vi "信号光谱6.vi"() -> ()   [LabVIEW 2018]
uses:
  <vilib>/Utility/NIReport.llb/Report Type.ctl
  <vilib>/Utility/file.llb/Write Delimited Spreadsheet (DBL).vi
  <vilib>/Instr/_visa.llb/VISA Configure Serial Port (Instr).vi
  <vilib>/addons/_office/excel.llb/Excel Get Data ([str]).vi
  <vilib>/Utility/NIReport.llb/NI_report.lvclass
  <vilib>/Analysis/NI_AALBase.lvlib
  <vilib>/ptbypt/NI_PtbyPt.lvlib
  <vilib>/Utility/NIReport.llb/NI_ReportGenerationCore.lvlib
  <vilib>/addons/_office/NI_ReportGenerationToolkit.lvlib
  <vilib>/Utility/NIReport.llb/Excel/NI_Excel.lvclass
panel:
  out "angle":dbl
  out "图片地址":string
  in  "开光时间/ms":u32=500
  out "最终存储路径 2":path
  out "照明光error out":errorcluster
  out "照明光":bool
  in  "stop bits (10: 1 bit)":u16(ring)=10 items=["1.0"=10, "1.5"=15, "2.0"=20]
  in  "parity (0:none)":enum16{"None", "Odd", "Even", "Mark", "Space"}(ring)
  in  "data bits (8)":u16=8 min=5 max=8 step=1
  in  "baud rate":u32=9600 caption="baud rate (115200)" min=9600 max=115200
  in  "VISA resource name":refnum<visa-resource-name>="COM7"
  out "正在测量":bool
  in  "滤波阈值":dbl=1500.0 format="%#_13g"
  out "best fit":dbl[][](graph) caption="最佳拟合"
  out "范围内？":bool[](array[boolean])
  out "w":dbl
  out "xc":dbl
  out "拟合参数":dbl[](array[numeric])
  out "最终存储路径":path
  in  "停止程序":bool
  in  "上升下降沿/s":dbl format="%.2p"
  in  "延时/s":dbl format="%.2p"
  in  "占空比/%":dbl=3.0 format="%.2p"
  in  "高电平/V":dbl=4.0 format="%.2p"
  in  "频率/Hz":dbl=6000.0 format="%.3p"
  in  "低电平/V":dbl min=0.0 max=5.0 format="%.2p"
  out "configure error out":errorcluster
  in  "设置参数":bool
  out "output control error  4":errorcluster
  in  "低电平持续输出":bool
  in  "Output 1":bool
  out "output control error  5":errorcluster
  in  "测量高电平/V":dbl=4.0
  out "output control error":errorcluster
  in  "开始测量":bool
  in  "上升下降沿":i32(ring)=1 items=["上升沿", "下降沿"]
  in  "channel输出口":i32(ring) items=["Channel 1", "Channel 2"]
  in  "输出信号波形":u16(ring) items=["Pulse"]
  out "output control error":errorcluster
  out "Output":bool
  in  "VISA 信号发生器":refnum<visa-resource-name>="USB0::0x1AB1::0x0641::DG4E192200870::INSTR"
  out "Spectrum":cluster{"Y":dbl[], "Y":dbl[]}[](graph)
  out "波长范围":dbl[](array[numeric])
  in  "选项卡控件":enum32{"IHR 550", "CCD"}(tab)
  in  "Move To\nTarget Positions":bool
  out "Current UniqueID":string="Mono4"
  in  "Mono ID":string(combo)="Mono1"
  in  "Connect":bool
  out "Initialized JY":bool=TRUE
  in  "Force\nInitialization":bool
  in  "Target Grating":string(combo)="2"
  out "Current Description":string="1" caption="Description"
  out "Grating Index":i32=1
  out "Current Grating":dbl=1200.0
  out "Units":string="nm"
  out "Current WL":dbl=897.9988
  out "Exit Mirror\nPosition":i32(ring)=2 items=["EntranceMirror", "ExitMirror", "Front", "Side"]
  out "Entrance Mirror\nPosition":i32(ring)=2 items=["EntranceMirror", "ExitMirror", "Front", "Side"]
  out "Units 2":string="mm"
  out "Front Entrance":dbl
  in  "Target WL":dbl=2670.0
  in  "Exit Mirror":u16(ring)=3 caption="Target Position Exit Mirror" items=["Front"=2, "Side"=3]
  in  "Entrance Mirror":u16(ring)=2 caption="Target Position\nEntrance Mirror" items=["Front"=2, "Side"=3]
  in  "Target\nFront Entrance":dbl=1.0
  in  "Commande tab":T1(tab)
  in  "Area Number to Display":i32
  in  "Reformat":bool
  in  "GAIN":u16(ring)=2 caption="Device Name" items=["High Light", "Best Dynamic Range", "High Sensitivity"]
  in  "ADC":u16(ring) caption="Device Name" items=["20 kHz       ", " 1 MHz       ", " 1 MHz Ultra "]
  in  "Number of Areas :":u16=1 min=1 step=1
  in  "Integration time (ms) :":i16=10000
  out "Uniques ID":u16(ring) items=["CCD1", "CCD2"]
  in  "Device Name":u16(ring) items=["Synapse CCD (Lateral)", "Synapse_IGA (Axial)"]
  in  "Signal type :":enum16{"TTL Rising Edge", "TTL Falling Edge"}(ring)=enum."TTL Falling Edge"
  in  "Trigger Type :":u16(ring) items=["On Start"=1, "Per Acquisition"=2]
  in  "trigSigTypeString":string
  in  "trigEventString":string
  in  "Enable InputTriggers :":bool
  in  "Number of Cleans":i32=1
  in  "MultiAcqShutterMode":i32(ring)=3 items=["Open For All Spectra"=1, "Open for Each Spectrum"=3]
  in  "Accumulations:":u16=10 min=1 step=1
  in  "Multi Accumulation mode:":bool
  out "Y Pixels:":i32=256
  out "DataSize":i32=1024
  out "X Pixels:":i32=1024
  out "Firmware\nVersion":string="V1.20 CCD_4000"
  out "initialized ?":bool=TRUE
  in  "Continuous":bool
  in  "CCD Busy":bool
  out "indicator":string="Ready !"
  in  "initialize":bool
  in  "ShutterOpen":bool=TRUE caption="Shutter enable"
  in  "Acquire":bool
  in  "Temperature":bool
  in  "Setup":bool
  out "Acq Time(ms)":u32=3401
  in  "Save Backlight":bool
  in  "cut backlight":bool
  out "backlight":bool=TRUE
  in  "是否拟合":bool
  in  "是否保存":bool
  in  "Close":bool=TRUE
  out "JYCCDLib.IJYCCDReqd":refnum<k7>
  out "areas :":i32[][](array[numeric])=[[1], [1], [1], [1024], [256], [1], [256]]
  in  "Constante de condition\n(Voir l'aide contextuelle)":bool
  out "temp graph":dbl(graph)=-134.538067
  out "ADC Number":i32[](array[numeric])=[0, 1, 2, 3, 4]
  out "Gain Number":i32[](array[numeric])=[10, 11, 12, 13, 8, 2]
  out "trigAddress":i32
  out "Data":i32[][](graph)
  out "error out":errorcluster
  out "Gratings":dbl[](array[numeric])=[1200.0, 300.0]
  out "Backlight":i32[][](graph)
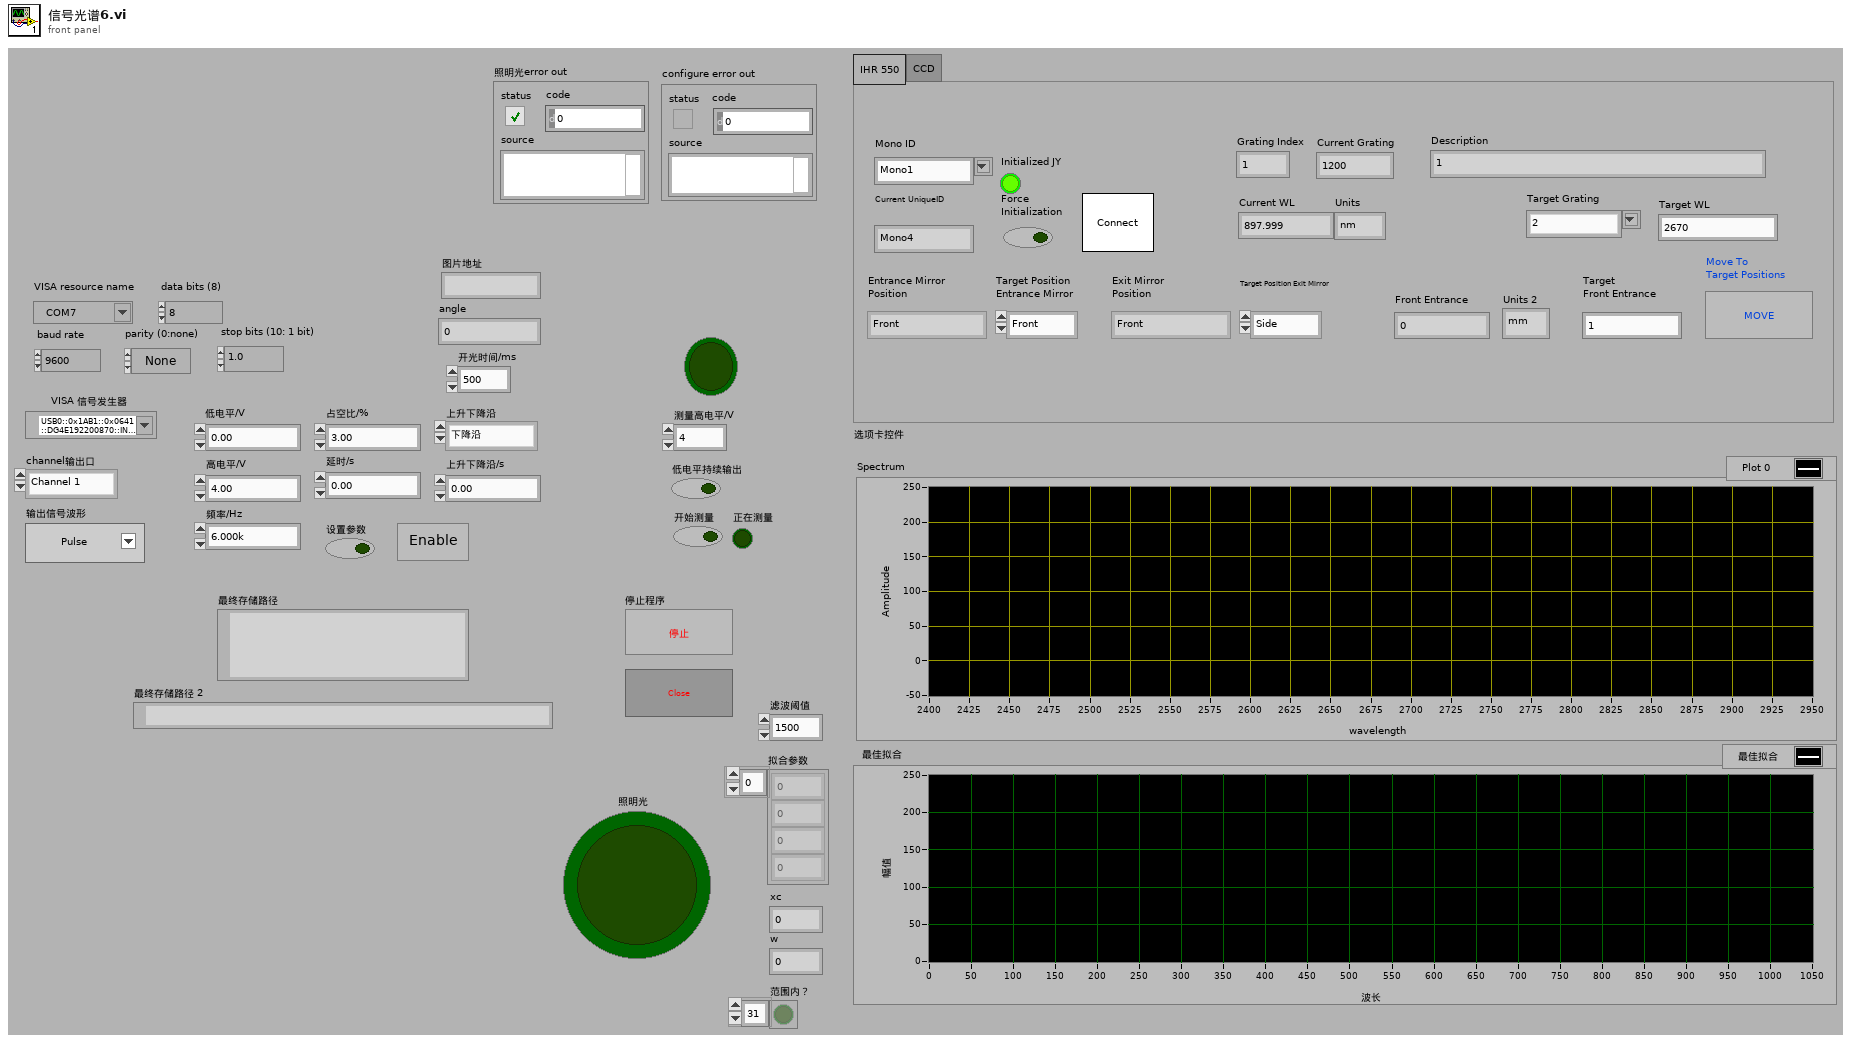
[diagram p1: front panel]
types:
  T1 = enum32{"Settings", "Trigger In", "Multi-Accu.", "Infos"}
  T2 = enum8{"Enabled", "Disabled", "Disabled and Grayed Out"}
  T3 = enum16{"maximized", "minimized", "normal", "no change"}
  T4 = typedef "NI_ReportGenerationCore.lvlib/Report Type.ctl" = enum16{"HTML", "Word", "Excel"}
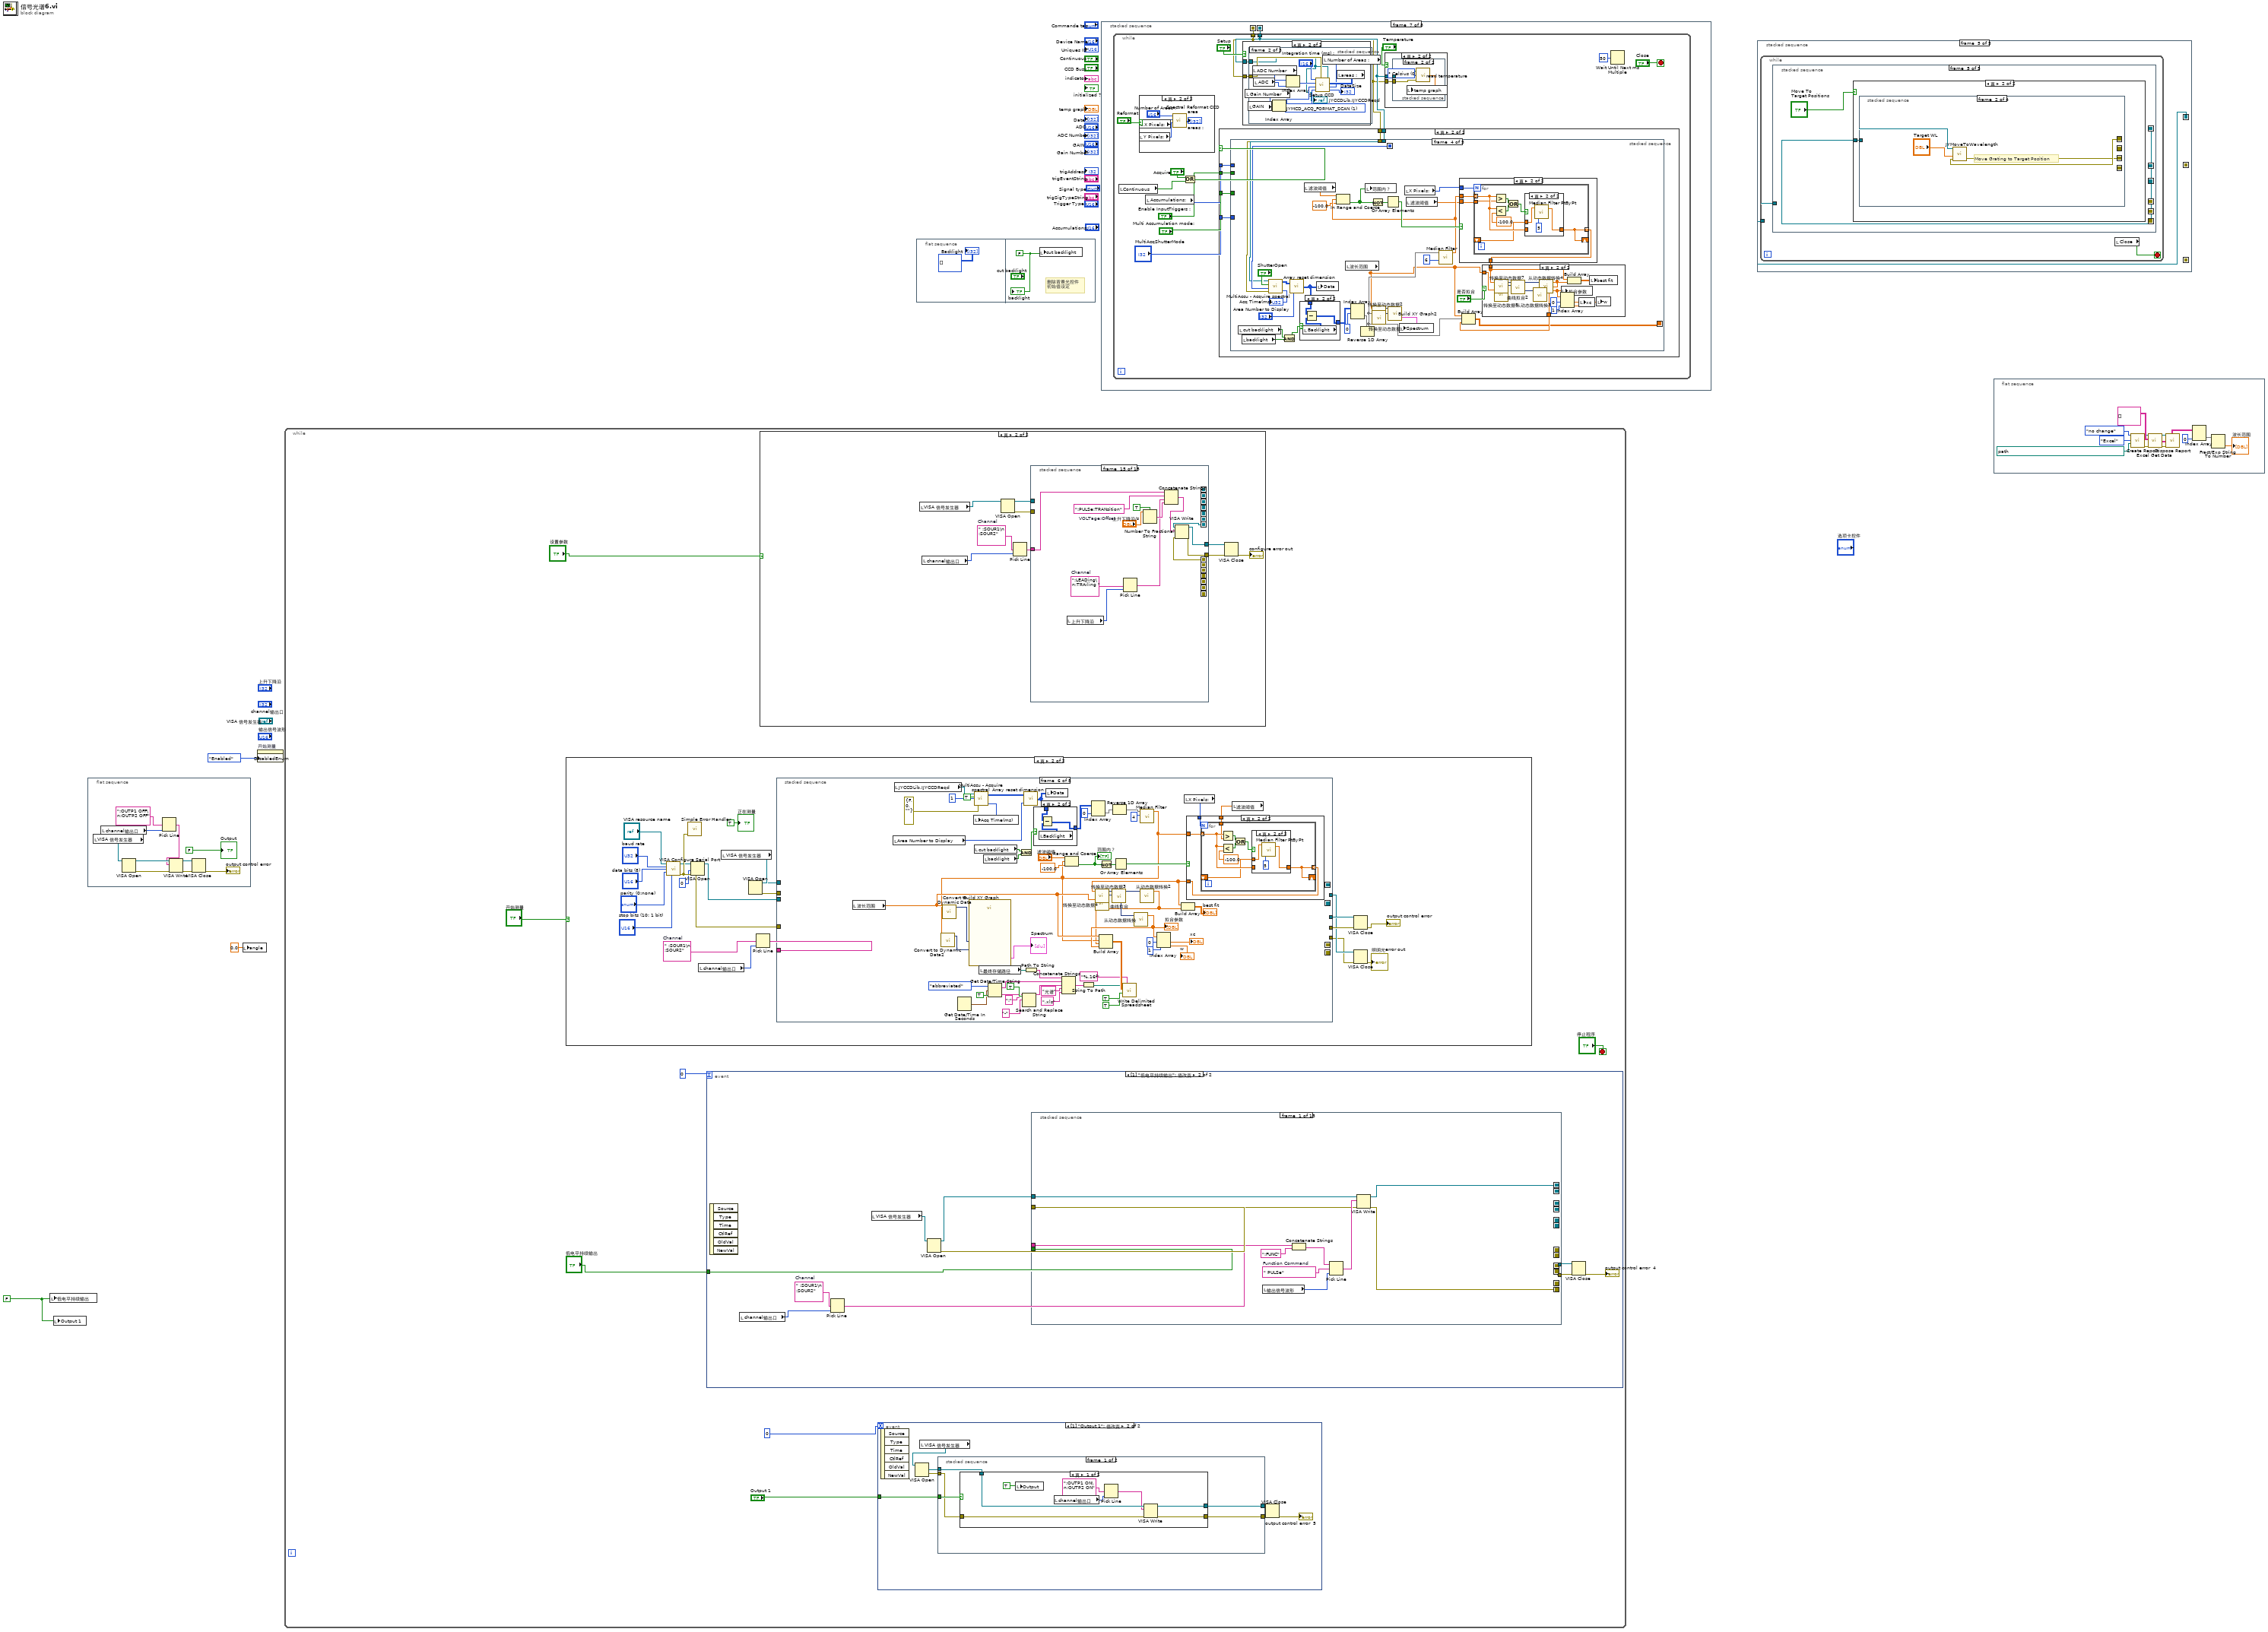
[diagram p0: block diagram]
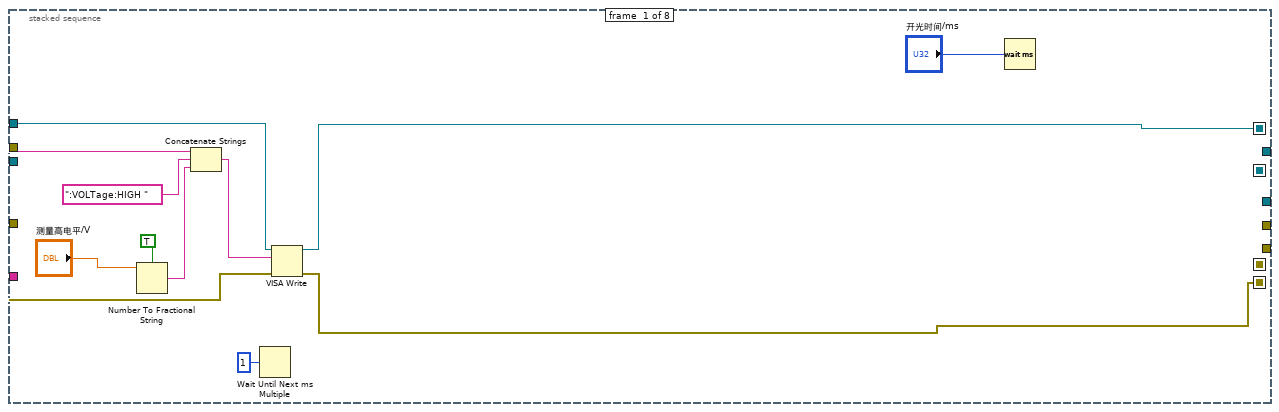
[diagram p3: hidden frame]
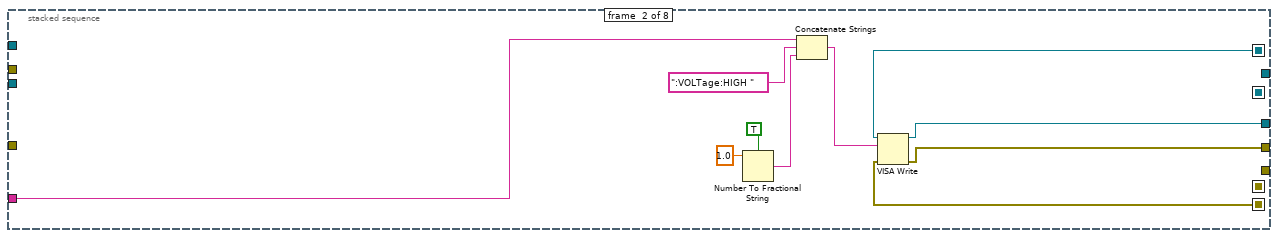
[diagram p4: hidden frame]
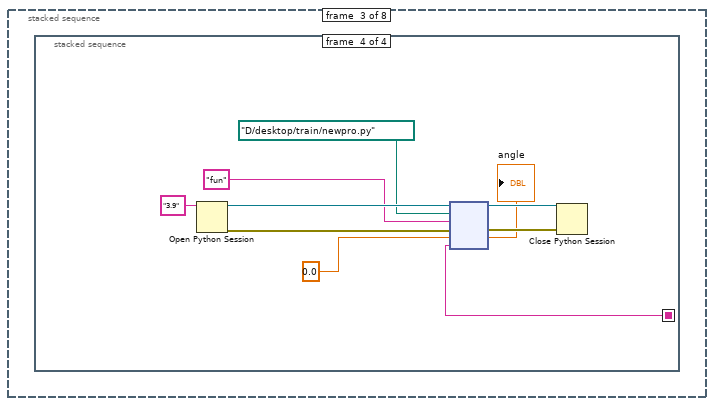
[diagram p5: hidden frame]
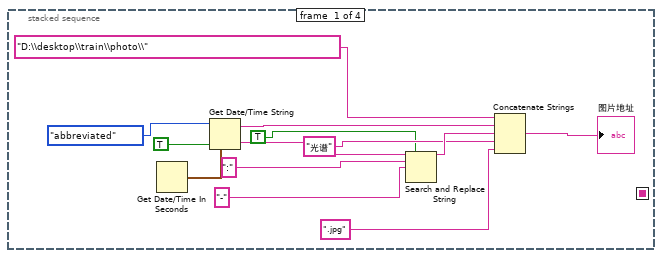
[diagram p6: hidden frame]
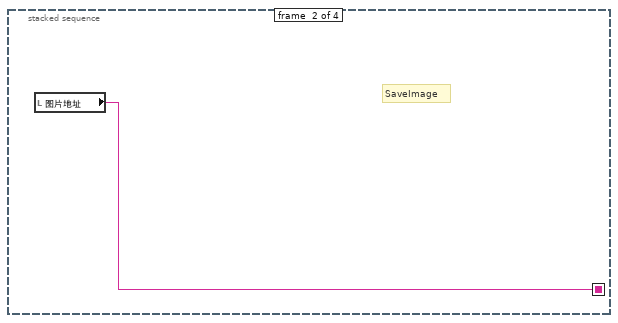
[diagram p7: hidden frame]
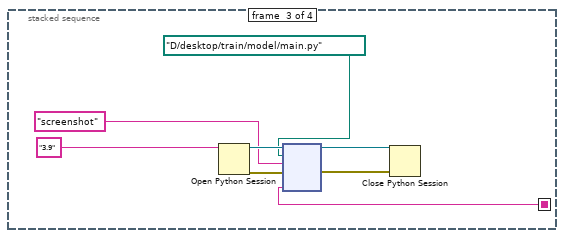
[diagram p8: hidden frame]
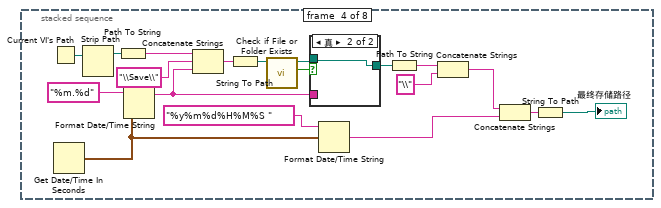
[diagram p9: hidden frame]
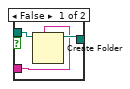
[diagram p10: hidden frame]
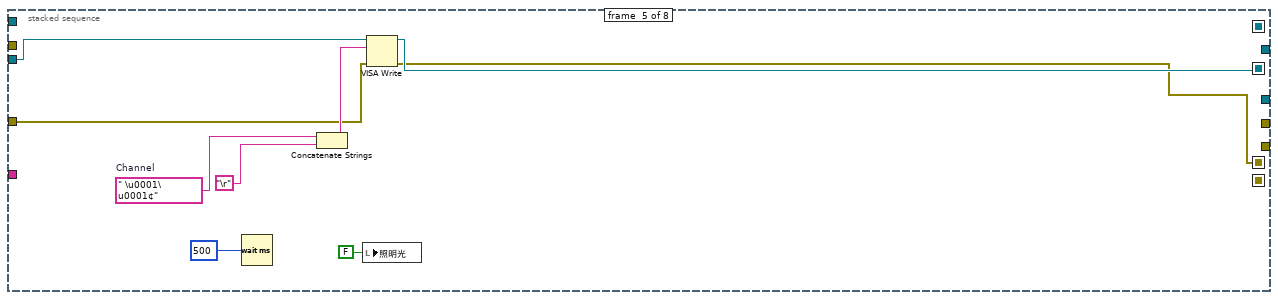
[diagram p11: hidden frame]
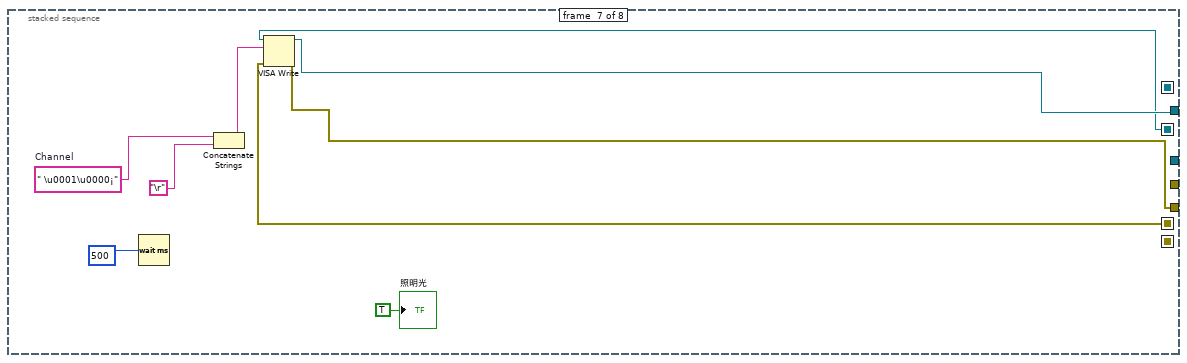
[diagram p15: hidden frame]
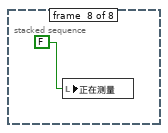
[diagram p16: hidden frame]
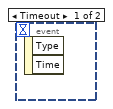
[diagram p17: hidden frame]
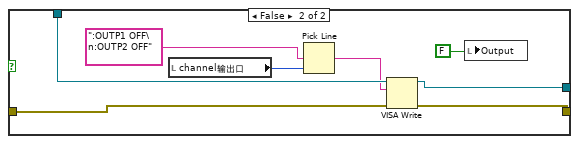
[diagram p18: hidden frame]
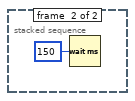
[diagram p19: hidden frame]
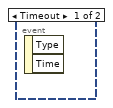
[diagram p20: hidden frame]
diagram:
  w2 = FALSE
  n1 = local write "低电平持续输出"(w2) -> ()
  n2 = local write "Output 1"(w2) -> ()
  n3 = flat-sequence {
    frame #0 {
      n4 = local read "VISA 信号发生器"() -> (w7:refnum<visa-resource-name>)
      n5 = local read "channel输出口"() -> (w5:i32)
      n6 = VISA Open(VISA resource name=w7) -> (VISA resource name=w13:refnum<visa-resource-name>, error out=w12:errorcluster)  [unwired: 4 in]
      n7 = Pick Line(multi-line string=":OUTP1 OFF\n:OUTP2 OFF" ("write buffer"), line index=w5) -> (output string=w4:string)  [unwired: 1 in]
      n8 = VISA Write(VISA resource name=w13, write buffer=w4, error in (no error)=w12) -> (VISA resource name out=w10:refnum<visa-resource-name>, error out=w9:errorcluster)  [unwired: 1 out]
      n9 = VISA Close(VISA resource name=w10, error in (no error)=w9) -> (error out=→"output control error":errorcluster)
      "Output" <- FALSE ("布尔")
    }
  }
  n10 = local write "angle"(0.0 ("angle")) -> ()
  n11 = property on="开始测量" class="Bool"("DisabledEnum"=T2."Enabled" ("禁用")) -> ()  [unwired: 2 in, 2 out]
  n12 = while {
    stop <- "停止程序" stop-if-true
    n13 = case shown="真" "开始测量" {
      frame False {
      }
      frame True {
        w36 = " :SOUR1\n :SOUR2"  # Channel
        n14 = call-poly "VISA Configure Serial Port"("VISA resource name"="VISA resource name", "baud rate (9600)"="baud rate", "data bits (8)"="data bits (8)", "parity (0:none)"="parity (0:none)", "stop bits (10: 1 bit)"="stop bits (10: 1 bit)") -> ("VISA resource name out"=w29:refnum<visa-resource-name>, "error out"=w30:errorcluster)  [unwired: 9 in]
        n15 = call <vilib>:"Simple Error Handler.vi"("error in (no error)"=w30) -> ()  [unwired: 4 in, 5 out]
        n16 = VISA Open(access mode=0, error in (no error)=w30, VISA resource name=w29) -> (VISA resource name=w22:refnum<visa-resource-name>, error out=w21:errorcluster)  [unwired: 2 in]
        n17 = local read "channel输出口"() -> (w37:i32)
        n18 = local read "VISA 信号发生器"() -> (w43:refnum<visa-resource-name>)
        n19 = VISA Open(VISA resource name=w43) -> (VISA resource name=w42:refnum<visa-resource-name>, error out=w41:errorcluster)  [unwired: 4 in]
        n20 = Pick Line(multi-line string=w36, line index=w37) -> (output string=w35:string)  [unwired: 1 in]
        n21 = stacked-sequence {
          seq-local: [w47 _ _ _ _ _ _ _] -> [_ w58 _ _ _ _ _ _]
          seq-local: [w46 _ _ _ _ _ _ _] -> [_ w57 _ _ _ _ _ _]
          seq-local: [_ _ _ _ w122 _ _ _] -> [_ _ _ _ _ _ w210 _]
          seq-local: [_ _ _ _ w121 _ _ _] -> [_ _ _ _ _ _ w213 _]
          tunnel: w42 -> [w50 _ _ _ _ _ _ _]
          tunnel: w41 -> [w49 _ _ _ _ _ _ _]
          tunnel: [_ w60 _ _ _ _ _ _] -> w40
          tunnel: [_ w59 _ _ _ _ _ _] -> w39
          tunnel: w35 -> [w51 w56 _ _ _ _ _ _]
          tunnel: w22 -> [_ _ _ _ w125 _ _ _]
          tunnel: w21 -> [_ _ _ _ w124 _ _ _]
          tunnel: [_ _ _ _ _ _ w212 _] -> w33
          tunnel: [_ _ _ _ _ _ w211 _] -> w32
          frame #0 {
            n22 = Number To Fractional String(use system decimal point (T)=TRUE ("使用系统小数点(T)"), number="测量高电平/V") -> (F-format string=w53:string)  [unwired: 2 in]
            n23 = Concatenate Strings ("连接字符串")(w51, ":VOLTage:HIGH ", w53) -> (w52:string)
            n24 = Wait Until Next ms Multiple(millisecond multiple=u32 1 ("毫秒倍数")) -> ()  [unwired: 1 out]
            n25 = VISA Write(VISA resource name=w50, write buffer=w52, error in (no error)=w49) -> (VISA resource name out=w47:refnum<visa-resource-name>, error out=w46:errorcluster)  [unwired: 1 out]
            n26 = Wait (ms)(milliseconds to wait="开光时间/ms") -> ()  [unwired: 1 out]
          }
          frame #1 {
            n27 = Number To Fractional String(use system decimal point (T)=TRUE ("使用系统小数点(T)"), number=1.0 ("数字")) -> (F-format string=w63:string)  [unwired: 2 in]
            n28 = Concatenate Strings ("连接字符串")(w56, ":VOLTage:HIGH ", w63) -> (w62:string)
            n29 = VISA Write(VISA resource name=w58, write buffer=w62, error in (no error)=w57) -> (VISA resource name out=w60:refnum<visa-resource-name>, error out=w59:errorcluster)  [unwired: 1 out]
          }
          frame #2 {
            n30 = stacked-sequence {
              seq-local: [_ w79 _ _] -> [_ _ w80 w88]
              frame #0 {
                n31 = Get Date/Time In Seconds() -> (seconds since 1Jan1904=w75:timestamp)
                n32 = Get Date/Time String(date format (0)=enum16{"short", "long", "abbreviated"}."abbreviated" ("日期格式(0)"), seconds (now)=w75, want seconds? (F)=TRUE ("需要秒？(F)")) -> (date string=w78:string, time string=w76:string)
                n33 = Search and Replace String(replace all?=TRUE ("替换全部？(F)"), input string=w76, search string=":" ("搜索字符串"), replace string="-" ("替换字符串(\"\")")) -> (result string=w77:string)  [unwired: 4 in, 3 out]
                n34 = Concatenate Strings("D:\\desktop\\train\\photo\\", w78, w77, "光谱" ("字符串"), ".jpg" ("字符串")) -> (→"图片地址":string)
              }
              frame #1 {
                # "SaveImage"
                n35 = local read "图片地址"() -> (w79:string)
              }
              frame #2 {
                n36 = Open Python Session(python version="3.9" ("Python version")) -> (session out=w87:refnum<k35>, error out=w85:errorcluster)  [unwired: 2 in]
                n37 = node(w87, path "D:/desktop/train/model/main.py" ("module path"), "screenshot" ("function name"), w85, w80) -> (w86:refnum<k35>, w84:errorcluster)  [unwired: 3 in, 2 out]
                n38 = Close Python Session(session in=w86, error in=w84) -> ()  [unwired: 1 out]
              }
              frame #3 {
                n39 = Open Python Session(python version="3.9" ("Python version")) -> (session out=w96:refnum<k35>, error out=w94:errorcluster)  [unwired: 2 in]
                n40 = node(w96, path "D:/desktop/train/newpro.py" ("module path"), "fun" ("function name"), w94, 0.0, w88) -> (w95:refnum<k35>, w93:errorcluster, →"angle":dbl)  [unwired: 1 in, 2 out]
                n41 = Close Python Session(session in=w95, error in=w93) -> ()  [unwired: 1 out]
              }
            }
          }
          frame #3 {
            n42 = Current VI's Path() -> (path=w103:path)
            n43 = Get Date/Time In Seconds() -> (seconds since 1Jan1904=w105:timestamp)
            n44 = Strip Path(path=w103) -> (stripped path=w104:path)  [unwired: 1 out]
            n45 = Path To String(path=w104) -> (string=w106:string)
            n46 = Format Date/Time String(time format string (%c)="%m.%d" ("时间格式字符串(%c)"), seconds (now)=w105) -> (date/time string=w112:string)  [unwired: 1 in]
            n47 = Concatenate Strings(w106, "\\Save\\" ("字符串"), w112) -> (w107:string)
            n48 = String To Path(string=w107) -> (path=w108:path)
            n49 = call <vilib>:"Check if File or Folder Exists.vi"("path"=w108) -> ("file or folder exists?"=w109:bool, "dup path"=w111:path)  [unwired: 8 in, 1 out]
            n50 = case shown="真" w109 {
              tunnel: [w119 w120] -> w110
              tunnel: w111 -> [w118 w120]
              tunnel: w112 -> [w117 _]
              frame False {
                n51 = Create Folder(prompt (Create Folder)=w117, path (use dialog)=w118) -> (created path=w119:path)  [unwired: 1 in, 2 out]
              }
              frame True {
              }
            }
            n52 = Format Date/Time String(time format string (%c)="%y%m%d%H%M%S " ("时间格式字符串(%c)"), seconds (now)=w105) -> (date/time string=w115:string)  [unwired: 1 in]
            n53 = Path To String(path=w110) -> (string=w113:string)
            n54 = Concatenate Strings(w113, "\\" ("字符串")) -> (w114:string)
            n55 = Concatenate Strings(w114, w115) -> (w102:string)
            n56 = String To Path(string=w102) -> (path=→"最终存储路径":path)
          }
          frame #4 {
            w126 = " \u0001\u0001¢"  # Channel
            n57 = Wait (ms)(milliseconds to wait=500) -> ()  [unwired: 1 out]
            n58 = Concatenate Strings(w126, "\r") -> (w127:string)
            n59 = local write "照明光"(FALSE ("照明光")) -> ()
            n60 = VISA Write(VISA resource name=w125, write buffer=w127, error in (no error)=w124) -> (VISA resource name out=w122:refnum<visa-resource-name>, error out=w121:errorcluster)  [unwired: 1 out]
          }
          frame #5 {
            n61 = local read "波长范围"() -> (w152:dbl[])
            n62 = local read "Area Number to Display"() -> (w162:i32)
            n63 = local read "JYCCDLib.IJYCCDReqd"() -> (w158:refnum<k7>)
            n64 = call "Convert to Dynamic Data"("Array"=w152) -> ("Dynamic Data Type"=w155:dynamicdata)  [unwired: 3 in]
            n65 = Get Date/Time In Seconds() -> (seconds since 1Jan1904=w171:timestamp)
            n66 = call "MultiAccu - Acquire spectral.vi"("error in"=errorcluster {"status"=FALSE, "code"=0, "source"=""}, "Accumulations:"=u16 1, "ShutterOpen"=TRUE, "JYCCDLib.IJYCCDReqd"=w158) -> ("Acq Time(ms)"=w164:u32, "Array Out"=w163:i32[][][])  [unwired: 1 out]
            n67 = local write "Acq Time(ms)"(w164) -> ()
            n68 = local read "cut backlight"() -> (w143:bool)
            n69 = local read "最终存储路径"() -> (w185:path)
            n70 = local read "backlight"() -> (w141:bool)
            n71 = Get Date/Time String(date format (0)=enum16{"short", "long", "abbreviated"}."abbreviated" ("日期格式(0)"), seconds (now)=w171, want seconds? (F)=TRUE ("需要秒？(F)")) -> (date string=w179:string, time string=w174:string)
            n72 = And(x=w143, y=w141) -> (x .and. y?=w142:bool)
            n73 = Search and Replace String(replace all?=TRUE ("替换全部？(F)"), input string=w174, search string=":" ("搜索字符串"), replace string="-" ("替换字符串(\"\")")) -> (result string=w178:string)  [unwired: 4 in, 3 out]
            n74 = call "Array reset dimension.vi"("Area Number"=w162, "Array In"=w163) -> ("Array Out"=w145:i32[][])
            n75 = Path To String(path=w185) -> (string=w168:string)
            n76 = case shown="真" w142 {
              tunnel: [w206 w208] -> w144
              tunnel: w145 -> [w206 w207]
              frame False {
              }
              frame True {
                n77 = local read "Backlight"() -> (w209:i32[][])
                n78 = Subtract(x=w207, y=w209) -> (x-y=w208:i32[][])
              }
            }
            n79 = local write "Data"(w145) -> ()
            n80 = Concatenate Strings(w168, w179, w178, "光谱" ("字符串"), ".xls" ("字符串")) -> (w183:string)
            n81 = String To Path(string=w183) -> (path=w184:path)
            n82 = Index Array(array=w144, index (row)=0 ("索引 (行)")) -> (element=w186:i32[])  [unwired: 1 in]
            n83 = call "转换至动态数据4"("Array"=w152) -> ("Dynamic Data Type"=w151:dynamicdata)  [unwired: 3 in]
            n84 = Reverse 1D Array(array=w186) -> (reversed array=w187:i32[])
            n85 = call <vilib>:"Median Filter.vi"("left rank"=4, "X"=w187) -> ("Filtered X"=w136:dbl[])  [unwired: 8 in, 1 out]
            n86 = call "Convert to Dynamic Data2"("Array"=w136) -> ("Dynamic Data Type"=w154:dynamicdata)  [unwired: 3 in]
            n87 = call "Build XY Graph"("Y Input"=w154, "X Input"=w155) -> ("XY Graph"=→"Spectrum":cluster{"Y":dbl[], "Y":dbl[]}[])  [unwired: 8 in, 1 out]
            n88 = In Range and Coerce(upper limit="滤波阈值", x=w136, lower limit=-100.0) -> (In Range?=w135:bool[])  [unwired: 1 out]
            "范围内？" <- w135
            n89 = Not(x=w135) -> (.not. x?=w134:bool[])
            n90 = Or Array Elements(Boolean array=w134) -> (logical OR=w138:bool)
            n91 = local read "X Pixels:"() -> (w137:i32)
            n92 = local read "滤波阈值"() -> (w130:dbl)
            n93 = case shown="真" w138 {
              tunnel: w137 -> [_ w193]
              tunnel: w136 -> [w189 w192]
              tunnel: [w189 w191] -> w133
              tunnel: w130 -> [_ w190]
              frame False {
              }
              frame True {
                n94 = for {
                  N: w193 -> [_]
                  tunnel: w192 -> [w197] mode=indexing
                  tunnel: [w196] -> w191 mode=indexing
                  shift-right: [w196] -> _
                  shift-left: _ -> [w195]
                  tunnel: w190 -> [w194]
                  n95 = Greater?(x=w197, y=w194) -> (0:w199:bool)
                  n96 = Less?(x=w197, y=-100.0) -> (x < y?=w200:bool)
                  n97 = Or(x=w199, y=w200) -> (x .or. y?=w198:bool)
                  n98 = case shown="真" w198 {
                    tunnel: w197 -> [w202 _]
                    tunnel: [w202 w204] -> w196
                    tunnel: w195 -> [_ w205]
                    frame False {
                    }
                    frame True {
                      n99 = call <vilib>:"Median Filter PtByPt.vi"("rank"=5, "x"=w205) -> ("Filtered x"=w204:dbl)  [unwired: 2 in, 1 out]
                    }
                  }
                }
              }
            }
            n100 = call "转换至动态数据3"("Array"=w133) -> ("Dynamic Data Type"=w153:dynamicdata)  [unwired: 3 in]
            n101 = call "曲线拟合"("Locations"=w151, "Signals"=w153) -> ("best fit"=w157:dynamicdata, "non-linear coefficients"=w156:dynamicdata)  [unwired: 5 in, 3 out]
            n102 = call "从动态数据转换"("Dynamic Data Type"=w156) -> ("Array"=w148:dbl[])  [unwired: 3 in]
            "拟合参数" <- w148
            n103 = call "从动态数据转换2"("Dynamic Data Type"=w157) -> ("Array"=w132:dbl[])  [unwired: 3 in]
            n104 = Build Array(w152, w136, w132, w148) -> (w188:dbl[][])
            n105 = call-poly <vilib>:"Write Delimited Spreadsheet.vi"("file path (dialog if empty)"=w184, "format (%.3f)"="%.16f", "2D data"=w188, "append to file? (new file:F)"=TRUE ("append to file? (F)"), "transpose? (no:F)"=TRUE ("transpose? (F)")) -> ()  [unwired: 9 in, 2 out]
            n106 = Index Array(array=w148, index #1=0 ("索引"), index #2=1 ("索引")) -> (element #1=→"xc":dbl, element #2=→"w":dbl)
            n107 = Build Array(w133, w132) -> (→"best fit":dbl[][])
          }
          frame #6 {
            w215 = " \u0001\u0000¡"  # Channel
            n108 = Wait (ms)(milliseconds to wait=500) -> ()  [unwired: 1 out]
            n109 = Concatenate Strings(w215, "\r") -> (w216:string)
            n110 = VISA Write(VISA resource name=w210, write buffer=w216, error in (no error)=w213) -> (VISA resource name out=w212:refnum<visa-resource-name>, error out=w211:errorcluster)  [unwired: 1 out]
            "照明光" <- TRUE ("照明光")
          }
          frame #7 {
            n111 = local write "正在测量"(FALSE) -> ()
          }
        }
        n112 = VISA Close(VISA resource name=w40, error in (no error)=w39) -> (error out=→"output control error":errorcluster)
        n113 = VISA Close(VISA resource name=w33, error in (no error)=w32) -> (error out=→"照明光error out":errorcluster)
        "正在测量" <- TRUE
      }
    }
    n114 = event shown="[1] \"低电平持续输出\": 值改变" {
      selector: _ -> [_ _]
      dyn-events: _ -> [_ _]
      timeout: u32 0 ("Time") -> [_ _]
      tunnel: "低电平持续输出" -> [_ w249]
      event Timeout {
        n115 = event-data() -> ()  [unwired: 1 in, 2 out]
      }
      event "低电平持续输出": Value Change {
        w253 = " :SOUR1\n :SOUR2"  # Channel
        n116 = event-data() -> ()  [unwired: 1 in, 6 out]
        n117 = local read "channel输出口"() -> (w254:i32)
        n118 = Pick Line(multi-line string=w253, line index=w254) -> (output string=w252:string)  [unwired: 1 in]
        n119 = local read "VISA 信号发生器"() -> (w257:refnum<visa-resource-name>)
        n120 = VISA Open(VISA resource name=w257) -> (VISA resource name=w256:refnum<visa-resource-name>, error out=w255:errorcluster)  [unwired: 4 in]
        n121 = stacked-sequence {
          seq-local: [w263 _ _ _ _ _ _ _ _ _ _ _ _] -> [_ _ w278 _ _ _ _ _ _ _ _ _ _]
          seq-local: [w262 _ _ _ _ _ _ _ _ _ _ _ _] -> [_ _ w277 _ _ _ _ _ _ _ _ _ _]
          seq-local: [_ _ w276 _ _ _ _ _ _ _ _ _ _] -> [_ _ _ _ w281 _ _ _ _ _ _ _ _]
          seq-local: [_ _ w275 _ _ _ _ _ _ _ _ _ _] -> [_ _ _ _ w282 _ _ _ _ _ _ _ _]
          seq-local: [_ _ _ _ w290 _ _ _ _ _ _ _ _] -> [_ _ _ _ _ _ w301 _ _ _ _ _ _]
          seq-local: [_ _ _ _ w289 _ _ _ _ _ _ _ _] -> [_ _ _ _ _ _ w300 _ _ _ _ _ _]
          seq-local: [_ _ _ _ _ _ w294 _ _ _ _ _ _] -> [_ _ _ _ _ _ _ _ w304 _ _ _ _]
          seq-local: [_ _ _ _ _ _ w293 _ _ _ _ _ _] -> [_ _ _ _ _ _ _ _ w303 _ _ _ _]
          seq-local: [_ _ _ _ _ _ _ _ w307 _ _ _ _] -> [_ _ _ _ _ _ _ _ _ _ w318 _ _]
          seq-local: [_ _ _ _ _ _ _ _ w306 _ _ _ _] -> [_ _ _ _ _ _ _ _ _ _ w317 _ _]
          seq-local: [_ _ _ _ _ _ _ _ _ _ w315 _ _] -> [_ _ _ _ _ _ _ _ _ _ _ _ w332]
          seq-local: [_ _ _ _ _ _ _ _ _ _ w314 _ _] -> [_ _ _ _ _ _ _ _ _ _ _ _ w331]
          tunnel: w256 -> [w268 _ _ _ _ _ _ _ _ _ _ _ _]
          tunnel: w255 -> [w261 _ _ _ _ _ _ _ _ _ _ _ _]
          tunnel: w252 -> [w260 _ w274 _ w287 _ w298 _ w308 _ w321 _ _]
          tunnel: [_ _ _ _ _ _ _ _ _ _ _ _ w330] -> w251
          tunnel: [_ _ _ _ _ _ _ _ _ _ _ _ w328] -> w250
          tunnel: w249 -> [_ _ _ _ _ _ _ _ _ _ _ _ w329]
          frame #0 {
            w265 = " PULSe"  # Function Command
            n122 = local read "输出信号波形"() -> (w259:u16)
            n123 = Concatenate Strings(w260, ":FUNC" ("string (\"\")")) -> (w266:string)
            n124 = Pick Line(string ("")=w266, multi-line string=w265, line index=w259) -> (output string=w264:string)
            n125 = VISA Write(VISA resource name=w268, write buffer=w264, error in (no error)=w261) -> (VISA resource name out=w263:refnum<visa-resource-name>, error out=w262:errorcluster)  [unwired: 1 out]
          }
          frame #1 {
            n126 = Wait (ms)(milliseconds to wait=u32 150) -> ()  [unwired: 1 out]
          }
          frame #2 {
            n127 = Number To Fractional String(use system decimal point (T)=TRUE ("使用系统小数点(T)"), number=1.0 ("数字")) -> (F-format string=w272:string)  [unwired: 2 in]
            n128 = Concatenate Strings ("连接字符串")(w274, ":VOLTage：HIGH ", w272) -> (w271:string)
            n129 = VISA Write(VISA resource name=w278, write buffer=w271, error in (no error)=w277) -> (VISA resource name out=w276:refnum<visa-resource-name>, error out=w275:errorcluster)  [unwired: 1 out]
          }
          frame #3 {
            n130 = Wait (ms)(milliseconds to wait=u32 150) -> ()  [unwired: 1 out]
          }
          frame #4 {
            # "1 电压偏置"
            n131 = Number To Fractional String(use system decimal point (T)=TRUE ("使用系统小数点(T)"), number=0.0 ("数字")) -> (F-format string=w285:string)  [unwired: 2 in]
            n132 = Concatenate Strings(w287, ":VOLTage:LOW ", w285) -> (w286:string)
            n133 = VISA Write(VISA resource name=w281, write buffer=w286, error in (no error)=w282) -> (VISA resource name out=w290:refnum<visa-resource-name>, error out=w289:errorcluster)  [unwired: 1 out]
          }
          frame #5 {
            n134 = Wait (ms)(milliseconds to wait=u32 150) -> ()  [unwired: 1 out]
          }
          frame #6 {
            n135 = local read "channel输出口"() -> (w296:i32)
            n136 = Pick Line(multi-line string=":OUTP1:IMPedance \n:OUTP2:IMPedance " ("write buffer"), line index=w296) -> (output string=w295:string)  [unwired: 1 in]
            n137 = Concatenate Strings ("连接字符串")(w298, w295, "INFINITY") -> (w299:string)
            n138 = VISA Write(VISA resource name=w301, write buffer=w299, error in (no error)=w300) -> (VISA resource name out=w294:refnum<visa-resource-name>, error out=w293:errorcluster)  [unwired: 1 out]
          }
          frame #7 {
            n139 = Wait (ms)(milliseconds to wait=u32 150) -> ()  [unwired: 1 out]
          }
          frame #8 {
            n140 = Number To Fractional String(use system decimal point (T)=TRUE ("使用系统小数点(T)"), number=0.0 ("数字")) -> (F-format string=w311:string)  [unwired: 2 in]
            n141 = Concatenate Strings(w308, ":PULSe:DELay ", w311) -> (w309:string)
            n142 = VISA Write(VISA resource name=w304, write buffer=w309, error in (no error)=w303) -> (VISA resource name out=w307:refnum<visa-resource-name>, error out=w306:errorcluster)  [unwired: 1 out]
          }
          frame #9 {
            n143 = Wait (ms)(milliseconds to wait=u32 150) -> ()  [unwired: 1 out]
          }
          frame #10 {
            w322 = ":LEADing\n:TRAiling "  # Channel
            w326 = ":PULSe:TRANsition"  # VOLTage:Offset
            n144 = local read "上升下降沿"() -> (w323:i32)
            n145 = Pick Line(multi-line string=w322, line index=w323) -> (output string=w319:string)  [unwired: 1 in]
            n146 = Number To Fractional String(use system decimal point (T)=TRUE ("使用系统小数点(T)"), number=0.0 ("数字")) -> (F-format string=w320:string)  [unwired: 2 in]
            n147 = Concatenate Strings(w321, w326, w319, w320) -> (w324:string)
            n148 = VISA Write(VISA resource name=w318, write buffer=w324, error in (no error)=w317) -> (VISA resource name out=w315:refnum<visa-resource-name>, error out=w314:errorcluster)  [unwired: 1 out]
          }
          frame #11 {
            n149 = Wait (ms)(milliseconds to wait=u32 150) -> ()  [unwired: 1 out]
          }
          frame #12 {
            n150 = case shown="假" w329 {
              tunnel: w332 -> [w340 w341]
              tunnel: [w339 w348] -> w328
              tunnel: w331 -> [w338 w346]
              tunnel: [w337 w347] -> w330
              frame True {
                n151 = local write "Output"(TRUE ("布尔")) -> ()
                n152 = local read "channel输出口"() -> (w334:i32)
                n153 = Pick Line(multi-line string=":OUTP1 ON\n:OUTP2 ON" ("write buffer"), line index=w334) -> (output string=w333:string)  [unwired: 1 in]
                n154 = VISA Write(VISA resource name=w340, write buffer=w333, error in (no error)=w338) -> (VISA resource name out=w337:refnum<visa-resource-name>, error out=w339:errorcluster)  [unwired: 1 out]
              }
              frame False {
                n155 = local read "channel输出口"() -> (w343:i32)
                n156 = Pick Line(multi-line string=":OUTP1 OFF\n:OUTP2 OFF" ("write buffer"), line index=w343) -> (output string=w342:string)  [unwired: 1 in]
                n157 = VISA Write(VISA resource name=w341, write buffer=w342, error in (no error)=w346) -> (VISA resource name out=w347:refnum<visa-resource-name>, error out=w348:errorcluster)  [unwired: 1 out]
                n158 = local write "Output"(FALSE ("布尔")) -> ()
              }
            }
          }
        }
        n159 = VISA Close(VISA resource name=w251, error in (no error)=w250) -> (error out=→"output control error  4":errorcluster)
      }
    }
    n160 = case shown="真" "设置参数" {
      frame False {
      }
      frame True {
        w354 = " :SOUR1\n :SOUR2"  # Channel
        n161 = local read "VISA 信号发生器"() -> (w350:refnum<visa-resource-name>)
        n162 = local read "channel输出口"() -> (w349:i32)
        n163 = VISA Open(VISA resource name=w350) -> (VISA resource name=w356:refnum<visa-resource-name>, error out=w357:errorcluster)  [unwired: 4 in]
        n164 = Pick Line(multi-line string=w354, line index=w349) -> (output string=w353:string)  [unwired: 1 in]
        n165 = stacked-sequence {
          seq-local: [w362 _ _ _ _ _ _ _ _ _ _ _ _ _ _] -> [_ _ w377 _ _ _ _ _ _ _ _ _ _ _ _]
          seq-local: [w361 _ _ _ _ _ _ _ _ _ _ _ _ _ _] -> [_ _ w376 _ _ _ _ _ _ _ w415 _ _ _ _]
          seq-local: [_ _ w375 _ _ _ _ _ _ _ _ _ _ _ _] -> [_ _ _ _ w386 _ _ _ _ _ _ _ _ _ _]
          seq-local: [_ _ w374 _ _ _ _ _ _ _ _ _ _ _ _] -> [_ _ _ _ w385 _ _ _ _ _ _ _ _ _ _]
          seq-local: [_ _ _ _ w384 _ _ _ _ _ _ _ _ _ _] -> [_ _ _ _ _ _ w392 _ _ _ _ _ _ _ _]
          seq-local: [_ _ _ _ w381 _ _ _ _ _ _ _ _ _ _] -> [_ _ _ _ _ _ w391 _ _ _ _ _ _ _ _]
          seq-local: [_ _ _ _ _ _ w399 _ _ _ _ _ _ _ _] -> [_ _ _ _ _ _ _ _ w410 _ _ _ _ _ _]
          seq-local: [_ _ _ _ _ _ w398 _ _ _ _ _ _ _ _] -> [_ _ _ _ _ _ _ _ w409 _ _ _ _ _ _]
          seq-local: [_ _ _ _ _ _ _ _ w403 _ _ _ _ _ _] -> [_ _ _ _ _ _ _ _ _ _ w416 _ _ _ _]
          seq-local: [_ _ _ _ _ _ _ _ w402 _ _ _ _ _ _] -> [_ _ _ _ _ _ _ _ _ _ _ _ _ _ _]
          seq-local: [_ _ _ _ _ _ _ _ _ _ w412 _ _ _ _] -> [_ _ _ _ _ _ _ _ _ _ _ _ w426 _ _]
          seq-local: [_ _ _ _ _ _ _ _ _ _ w413 _ _ _ _] -> [_ _ _ _ _ _ _ _ _ _ _ _ w425 _ _]
          seq-local: [_ _ _ _ _ _ _ _ _ _ _ _ w424 _ _] -> [_ _ _ _ _ _ _ _ _ _ _ _ _ _ w437]
          seq-local: [_ _ _ _ _ _ _ _ _ _ _ _ w423 _ _] -> [_ _ _ _ _ _ _ _ _ _ _ _ _ _ w436]
          tunnel: w356 -> [w367 _ _ _ _ _ _ _ _ _ _ _ _ _ _]
          tunnel: w357 -> [w360 _ _ _ _ _ _ _ _ _ _ _ _ _ _]
          tunnel: w353 -> [w359 _ w373 _ w380 _ w396 _ w407 _ w417 _ w427 _ w440]
          tunnel: [_ _ _ _ _ _ _ _ _ _ _ _ _ _ w435] -> w352
          tunnel: [_ _ _ _ _ _ _ _ _ _ _ _ _ _ w434] -> w351
          frame #0 {
            w364 = " PULSe"  # Function Command
            n166 = local read "输出信号波形"() -> (w358:u16)
            n167 = Concatenate Strings(w359, ":FUNC" ("string (\"\")")) -> (w365:string)
            n168 = Pick Line(string ("")=w365, multi-line string=w364, line index=w358) -> (output string=w363:string)
            n169 = VISA Write(VISA resource name=w367, write buffer=w363, error in (no error)=w360) -> (VISA resource name out=w362:refnum<visa-resource-name>, error out=w361:errorcluster)  [unwired: 1 out]
          }
          frame #1 {
            n170 = Wait (ms)(milliseconds to wait=u32 150) -> ()  [unwired: 1 out]
          }
          frame #2 {
            n171 = Number To Fractional String(use system decimal point (T)=TRUE ("使用系统小数点(T)"), number="低电平/V") -> (F-format string=w371:string)  [unwired: 2 in]
            n172 = Concatenate Strings ("连接字符串")(w373, ":VOLTage:LOW ", w371) -> (w370:string)
            n173 = VISA Write(VISA resource name=w377, write buffer=w370, error in (no error)=w376) -> (VISA resource name out=w375:refnum<visa-resource-name>, error out=w374:errorcluster)  [unwired: 1 out]
          }
          frame #3 {
            n174 = Wait (ms)(milliseconds to wait=u32 150) -> ()  [unwired: 1 out]
          }
          frame #4 {
            # "1 频率"
            n175 = Concatenate Strings(w380, ":FREQ ") -> (w387:string)
            n176 = Format Into String ("格式化写入字符串")(initial string=w387, "频率/Hz") -> (resulting string=w388:string)  [unwired: 2 in, 1 out]
            n177 = VISA Write(VISA resource name=w386, write buffer=w388, error in (no error)=w385) -> (VISA resource name out=w384:refnum<visa-resource-name>, error out=w381:errorcluster)  [unwired: 1 out]
          }
          frame #5 {
            n178 = Wait (ms)(milliseconds to wait=u32 150) -> ()  [unwired: 1 out]
          }
          frame #6 {
            n179 = Number To Fractional String(use system decimal point (T)=TRUE ("使用系统小数点(T)"), number="高电平/V") -> (F-format string=w393:string)  [unwired: 2 in]
            n180 = Concatenate Strings(w396, ":VOLTage:HIGH ", w393) -> (w395:string)
            n181 = VISA Write(VISA resource name=w392, write buffer=w395, error in (no error)=w391) -> (VISA resource name out=w399:refnum<visa-resource-name>, error out=w398:errorcluster)  [unwired: 1 out]
          }
          frame #7 {
            n182 = Wait (ms)(milliseconds to wait=u32 150) -> ()  [unwired: 1 out]
          }
          frame #8 {
            n183 = local read "channel输出口"() -> (w405:i32)
            n184 = Pick Line(multi-line string=":OUTP1:IMPedance \n:OUTP2:IMPedance " ("write buffer"), line index=w405) -> (output string=w404:string)  [unwired: 1 in]
            n185 = Concatenate Strings ("连接字符串")(w407, w404, "INFINITY") -> (w408:string)
            n186 = VISA Write(VISA resource name=w410, write buffer=w408, error in (no error)=w409) -> (VISA resource name out=w403:refnum<visa-resource-name>, error out=w402:errorcluster)  [unwired: 1 out]
          }
          frame #9 {
            n187 = Wait (ms)(milliseconds to wait=u32 150) -> ()  [unwired: 1 out]
          }
          frame #10 {
            n188 = Number To Fractional String(use system decimal point (T)=TRUE ("使用系统小数点(T)"), number="占空比/%") -> (F-format string=w419:string)  [unwired: 2 in]
            n189 = Concatenate Strings(w417, ":PULSe:DCYCle ", w419) -> (w414:string)
            n190 = VISA Write(VISA resource name=w416, write buffer=w414, error in (no error)=w415) -> (VISA resource name out=w412:refnum<visa-resource-name>, error out=w413:errorcluster)  [unwired: 1 out]
          }
          frame #11 {
            n191 = Wait (ms)(milliseconds to wait=u32 150) -> ()  [unwired: 1 out]
          }
          frame #12 {
            n192 = Number To Fractional String(use system decimal point (T)=TRUE ("使用系统小数点(T)"), number="延时/s") -> (F-format string=w430:string)  [unwired: 2 in]
            n193 = Concatenate Strings(w427, ":PULSe:DELay ", w430) -> (w428:string)
            n194 = VISA Write(VISA resource name=w426, write buffer=w428, error in (no error)=w425) -> (VISA resource name out=w424:refnum<visa-resource-name>, error out=w423:errorcluster)  [unwired: 1 out]
          }
          frame #13 {
            n195 = Wait (ms)(milliseconds to wait=u32 150) -> ()  [unwired: 1 out]
          }
          frame #14 {
            w441 = ":LEADing\n:TRAiling "  # Channel
            w446 = ":PULSe:TRANsition"  # VOLTage:Offset
            n196 = local read "上升下降沿"() -> (w442:i32)
            n197 = Pick Line(multi-line string=w441, line index=w442) -> (output string=w438:string)  [unwired: 1 in]
            n198 = Number To Fractional String(use system decimal point (T)=TRUE ("使用系统小数点(T)"), number="上升下降沿/s") -> (F-format string=w439:string)  [unwired: 2 in]
            n199 = Concatenate Strings(w440, w446, w438, w439) -> (w443:string)
            n200 = VISA Write(VISA resource name=w437, write buffer=w443, error in (no error)=w436) -> (VISA resource name out=w435:refnum<visa-resource-name>, error out=w434:errorcluster)  [unwired: 1 out]
          }
        }
        n201 = VISA Close(VISA resource name=w352, error in (no error)=w351) -> (error out=→"configure error out":errorcluster)
      }
    }
    n202 = event shown="[1] \"Output 1\": 值改变" {
      selector: _ -> [_ _]
      dyn-events: _ -> [_ _]
      timeout: u32 0 ("Time") -> [_ _]
      tunnel: "Output 1" -> [_ w224]
      event Timeout {
        n203 = event-data() -> ()  [unwired: 1 in, 2 out]
      }
      event "Output 1": Value Change {
        n204 = event-data() -> ()  [unwired: 1 in, 6 out]
        n205 = local read "VISA 信号发生器"() -> (w220:refnum<visa-resource-name>)
        n206 = VISA Open(VISA resource name=w220) -> (VISA resource name=w223:refnum<visa-resource-name>, error out=w226:errorcluster)  [unwired: 4 in]
        n207 = stacked-sequence {
          tunnel: w224 -> [w231 _]
          tunnel: w226 -> [w230 _]
          tunnel: w223 -> [w229 _]
          tunnel: [w228 _] -> w222
          tunnel: [w227 _] -> w221
          frame #0 {
            n208 = case shown="真" w231 {
              tunnel: w229 -> [w239 w247]
              tunnel: [w238 w246] -> w227
              tunnel: w230 -> [w237 w244]
              tunnel: [w236 w245] -> w228
              frame True {
                n209 = local write "Output"(TRUE ("布尔")) -> ()
                n210 = local read "channel输出口"() -> (w233:i32)
                n211 = Pick Line(multi-line string=":OUTP1 ON\n:OUTP2 ON" ("write buffer"), line index=w233) -> (output string=w232:string)  [unwired: 1 in]
                n212 = VISA Write(VISA resource name=w239, write buffer=w232, error in (no error)=w237) -> (VISA resource name out=w236:refnum<visa-resource-name>, error out=w238:errorcluster)  [unwired: 1 out]
              }
              frame False {
                n213 = local read "channel输出口"() -> (w241:i32)
                n214 = Pick Line(multi-line string=":OUTP1 OFF\n:OUTP2 OFF" ("write buffer"), line index=w241) -> (output string=w240:string)  [unwired: 1 in]
                n215 = VISA Write(VISA resource name=w247, write buffer=w240, error in (no error)=w244) -> (VISA resource name out=w245:refnum<visa-resource-name>, error out=w246:errorcluster)  [unwired: 1 out]
                n216 = local write "Output"(FALSE ("布尔")) -> ()
              }
            }
          }
          frame #1 {
            n217 = Wait (ms)(milliseconds to wait=u32 150) -> ()  [unwired: 1 out]
          }
        }
        n218 = VISA Close(VISA resource name=w222, error in (no error)=w221) -> (error out=→"output control error  5":errorcluster)
      }
    }
  }
  n219 = flat-sequence {
    frame #0 {
      "Backlight" <- i32[][] [] ("Backlight")
    }
    frame #1 {
      w448 = FALSE
      # "删除背景光控件\n初始值设定"
      n220 = local write "cut backlight"(w448) -> ()
      "backlight" <- w448
    }
  }
  n221 = stacked-sequence {
    seq-local: [_ _ _ w469 _ _ _ _] -> [_ _ _ _ w487 w507 w510 w703]
    seq-local: [_ _ _ w468 _ _ _ _] -> [_ _ _ _ w488 w508 w509 w704]
    frame #0 {
      # "initialize all variables"
      n222 = property on="initialize" class="Bool"("Désactivé"=u8 0) -> ()  [unwired: 2 in, 2 out]
      n223 = property on="Acquire" class="Bool"("Visible"=FALSE) -> ()  [unwired: 2 in, 2 out]
      n224 = property on="Setup" class="Bool"("Visible"=FALSE) -> ()  [unwired: 2 in, 2 out]
      n225 = local write "indicator"("" ("indicator")) -> ()
      n226 = local write "initialized ?"(FALSE ("initialized ?")) -> ()
      n227 = local write "Continuous"(FALSE ("Continuous")) -> ()
      n228 = local write "Close"(FALSE ("Close")) -> ()
      n229 = property on="Device Name" class="Ring (严格)"("Désactivé"=u8 0) -> ()  [unwired: 2 in, 2 out]
      n230 = property on="Continuous" class="Bool (严格)"("Visible"=FALSE) -> ()  [unwired: 2 in, 2 out]
      n231 = local write "Commande tab"(T1."Settings" ("Commande tab")) -> ()
    }
    frame #1 {
      # "Read Uniq ID"
      n232 = stacked-sequence {
        frame #0 {
          n233 = call "read detector uniq-id.vi"() -> ("nbr of components"=w461:i32, "UniqueID"=w460:string[], "Name"=w459:string[])  [unwired: 4 out]
          n234 = for {
            N: w461 -> [_]
            tunnel: w460 -> [w463]
            tunnel: w459 -> [w462]
            n235 = property on="Device Name" class="Ring (严格)"("Chaînes []"=w462) -> ()  [unwired: 2 in, 2 out]
            n236 = property on="Uniques ID" class="Ring (严格)"("Chaînes []"=w463) -> ()  [unwired: 2 in, 2 out]
          }
        }
      }
    }
    frame #2 {
      n237 = while {
        stop <- "initialize" stop-if-true
        n238 = local read "Device Name"() -> (w466:u16)
        n239 = local write "Uniques ID"(w466) -> ()
        n240 = local read "Close"() -> (w464:bool)
        n241 = Stop(stop? (T)=w464) -> ()
        n242 = Wait Until Next ms Multiple(millisecond multiple=u32 100 ("n millisecondes")) -> ()  [unwired: 1 out]
      }
    }
    frame #3 {
      n243 = stacked-sequence {
        tunnel: [_ w476 _ _] -> w469
        tunnel: [_ w475 _ _] -> w468
        frame #0 {
          n244 = local write "indicator"("Initializing ..." ("indicator")) -> ()
        }
        frame #1 {
          n245 = local read "Uniques ID"() -> (w473:u16)
          n246 = property on="Uniques ID" class="Ring (严格)"() -> ("Chaînes []"=w474:string[])  [unwired: 2 in, 2 out]
          n247 = Index Array(array=w474, index=w473) -> (element=w472:string)
          n248 = call "Initialize CCD.vi"("Unique id:"=w472) -> ("activeYPixels"=→"Y Pixels:":i32, "JYCCDLib.IJYCCDReqd"=w475:refnum<k7>, "activeXPixels"=→"X Pixels:":i32, "sortie d'erreur"=w476:errorcluster, "FirmwareVersion"=→"Firmware\nVersion":string)  [unwired: 3 out]
        }
        frame #2 {
          n249 = property on="initialize" class="Bool"("Désactivé"=u8 2) -> ()  [unwired: 2 in, 2 out]
          n250 = property on="Device Name" class="Ring (严格)"("Désactivé"=u8 2) -> ()  [unwired: 2 in, 2 out]
          n251 = local write "Continuous"(FALSE ("Continuous")) -> ()
          n252 = property on="Setup" class="Bool"("Visible"=TRUE) -> ()  [unwired: 2 in, 2 out]
        }
        frame #3 {
          n253 = local write "initialized ?"(TRUE ("initialized ?")) -> ()
          n254 = local write "indicator"("Initialized !" ("indicator")) -> ()
        }
      }
    }
    frame #4 {
      # "Actually not working"
      # "Read ADC and GAIN"
      n255 = case shown="真" "Constante de condition\n(Voir l'aide contextuelle)" {
        tunnel: w488 -> [_ w498]
        tunnel: w487 -> [_ w497]
        frame False {
        }
        frame True {
          # "Read Input supported trigger"
          n256 = call "Trigger - Get Supported Input.vi"("JYCCDLib.IJYCCDReqd"=w498, "Error Input"=w497) -> ("trigAddress"=w492:i32, "eventPtr"=w493:i32, "trigEventString"=w496:string, "trigSigType"=w495:i32, "trigSigTypeString"=w494:string)  [unwired: 4 out]
          n257 = local write "trigSigTypeString"(w494) -> ()
          n258 = local write "trigAddress"(w492) -> ()
          n259 = local write "Trigger Type :"(w493) -> ()
          n260 = local write "trigEventString"(w496) -> ()
          n261 = local write "Signal type :"(w495) -> ()
        }
      }
      n262 = call "Init ADC & Gain.vi"("JYCCDLib.IJYCCDReqd"=w488, "input error"=w487) -> ("ADC Number"=w486:i32[], "ADC description"=w491:string[], "Gain Number"=w489:i32[], "Gain description"=w490:string[])
      n263 = local write "Gain Number"(w489) -> ()
      n264 = local write "ADC Number"(w486) -> ()
      n265 = stacked-sequence {
        tunnel: w491 -> [w499 _]
        tunnel: w490 -> [_ w500]
        frame #0 {
          n266 = property on="ADC" class="Ring (严格)"("Chaînes []"=w499) -> ()  [unwired: 2 in, 2 out]
        }
        frame #1 {
          n267 = property on="GAIN" class="Ring (严格)"("Chaînes []"=w500) -> ()  [unwired: 2 in, 2 out]
        }
      }
    }
    frame #5 {
      # "IS multi Accumulation Supported ?"
      n268 = call "MultiAccu - Is Supported.vi"("Error In"=w507, "JYCCDLib.IJYCCDReqd"=w508) -> ("IsOperatingModeSupported"=w501:bool)  [unwired: 3 out]
      n269 = Select(t=0, s=w501, f=2) -> (s? t:f=w504:i32)
      n270 = Select(t=FALSE, s=w501, f=w501) -> (s? t:f=w503:bool)
      n271 = local write "Multi Accumulation mode:"(w503) -> ()
      n272 = property on="Multi Accumulation mode:" class="Bool (严格)"("Désactivé"=w504) -> ()  [unwired: 2 in, 2 out]
      n273 = property on="Multi Accumulation mode:" class="Bool (严格)"("Désactivé"=w504) -> ()  [unwired: 2 in, 2 out]
    }
    frame #6 {
      n274 = while {
        tunnel: w509 -> [w517]
        tunnel: w510 -> [w516]
        stop <- "Close" stop-if-true
        n275 = local read "Continuous"() -> (w518:bool)
        n276 = case shown="真" "Reformat" {
          frame False {
          }
          frame True {
            n277 = local read "Y Pixels:"() -> (w681:i32)
            n278 = local read "X Pixels:"() -> (w683:i32)
            n279 = call "Spectral Reformat CCD area.vi"("Y Pixels:"=w681, "X Pixels:"=w683, "numAreas"="Number of Areas :") -> ("areas :"=→"areas :":i32[][])  [unwired: 3 out]
          }
        }
        n280 = local read "Accumulations:"() -> (w513:u16)
        n281 = Or(x="Acquire", y=w518) -> (x .or. y?=w515:bool)
        n282 = case shown="真" w515 {
          tunnel: w517 -> [_ w530]
          tunnel: w516 -> [_ w529]
          tunnel: "Enable InputTriggers :" -> [_ w528]
          tunnel: "Multi Accumulation mode:" -> [_ w527]
          tunnel: w513 -> [_ w526]
          tunnel: "MultiAcqShutterMode" -> [_ w525]
          frame False {
          }
          frame True {
            n283 = stacked-sequence {
              seq-local: [_ _ w543 _ _] -> [_ _ _ w609 _]
              seq-local: [_ _ _ w580 _] -> [_ _ _ _ w647]
              tunnel: w530 -> [_ w532 w547 w608 _]
              tunnel: w529 -> [_ w533 w546 w607 _]
              tunnel: w528 -> [_ w534 _ _ _]
              tunnel: w527 -> [_ _ w545 _ _]
              tunnel: w526 -> [_ _ w544 _ _]
              tunnel: w525 -> [_ _ w542 _ _]
              frame #0 {
                n284 = local write "CCD Busy"(TRUE ("CCD Busy")) -> ()
              }
              frame #1 {
                n285 = case shown="真" w534 {
                  tunnel: w533 -> [w535 w541]
                  tunnel: w532 -> [w536 w540]
                  frame False {
                    n286 = call "Trigger - Disable.vi"("Error In"=w535, "JYCCDLib.IJYCCDReqd"=w536) -> ()  [unwired: 6 out]
                  }
                  frame True {
                    n287 = local read "Trigger Type :"() -> (w537:u16)
                    n288 = local read "Signal type :"() -> (w538:enum16{"TTL Rising Edge", "TTL Falling Edge"})
                    n289 = local read "trigAddress"() -> (w539:i32)
                    n290 = call "Trigger - Enable.vi"("Error In"=w541, "sigType"=w538, "event"=w537, "trigAddress"=w539, "JYCCDLib.IJYCCDReqd"=w540) -> ()  [unwired: 3 out]
                  }
                }
              }
              frame #2 {
                n291 = case shown="真" w545 {
                  selector: w545 -> [_ w576]
                  tunnel: w547 -> [w573 w579]
                  tunnel: w546 -> [w572 w578]
                  tunnel: w544 -> [_ w577]
                  tunnel: [u16 1 ("Accumulations:") w577] -> w543
                  tunnel: w542 -> [_ w575]
                  frame False {
                    n292 = call "MultiAccu - Disable.vi"("Error In"=w572, "JYCCDLib.IJYCCDReqd"=w573) -> ()  [unwired: 4 out]
                  }
                  frame True {
                    n293 = call "MultiAccu - Configure.vi"("JYCCDLib.IJYCCDReqd"=w579, "Cleans Before"="Number of Cleans", "Accumulations:"=w577, "MultiAcqHardwareMode"=w576, "MultiAcqShutterMode"=w575, "Error In"=w578) -> ()  [unwired: 1 in, 9 out]
                  }
                }
                n294 = flat-sequence {
                  frame #0 {
                    n295 = Current VI's Path() -> (path=w553:path)
                    n296 = Get Date/Time In Seconds() -> (seconds since 1Jan1904=w555:timestamp)
                    n297 = Strip Path(path=w553) -> (stripped path=w554:path)  [unwired: 1 out]
                    n298 = Path To String(path=w554) -> (string=w556:string)
                    n299 = Format Date/Time String(time format string (%c)="%m.%d" ("时间格式字符串(%c)"), seconds (now)=w555) -> (date/time string=w562:string)  [unwired: 1 in]
                    n300 = Concatenate Strings(w556, "\\Save\\" ("字符串"), w562) -> (w557:string)
                    n301 = String To Path(string=w557) -> (path=w558:path)
                    n302 = call <vilib>:"Check if File or Folder Exists.vi"("path"=w558) -> ("file or folder exists?"=w559:bool, "dup path"=w561:path)  [unwired: 8 in, 1 out]
                    n303 = case shown="真" w559 {
                      tunnel: [w569 w570] -> w560
                      tunnel: w561 -> [w568 w570]
                      tunnel: w562 -> [w567 _]
                      frame False {
                        n304 = Create Folder(prompt (Create Folder)=w567, path (use dialog)=w568) -> (created path=w569:path)  [unwired: 1 in, 2 out]
                      }
                      frame True {
                      }
                    }
                    n305 = Format Date/Time String(time format string (%c)="%y%m%d%H%M%S " ("时间格式字符串(%c)"), seconds (now)=w555) -> (date/time string=w565:string)  [unwired: 1 in]
                    n306 = Path To String(path=w560) -> (string=w563:string)
                    n307 = Concatenate Strings(w563, "\\" ("字符串")) -> (w564:string)
                    n308 = Concatenate Strings(w564, w565) -> (w552:string)
                    n309 = String To Path(string=w552) -> (path=→"最终存储路径 2":path)
                  }
                }
              }
              frame #3 {
                n310 = local read "cut backlight"() -> (w596:bool)
                n311 = local read "backlight"() -> (w595:bool)
                n312 = call "MultiAccu - Acquire spectral.vi"("error in"=w607, "Accumulations:"=w609, "ShutterOpen"="ShutterOpen", "JYCCDLib.IJYCCDReqd"=w608) -> ("Acq Time(ms)"=→"Acq Time(ms)":u32, "Array Out"=w606:i32[][][])  [unwired: 1 out]
                n313 = And(x=w596, y=w595) -> (x .and. y?=w597:bool)
                n314 = call "Array reset dimension.vi"("Area Number"="Area Number to Display", "Array In"=w606) -> ("Array Out"=w598:i32[][])
                n315 = case shown="真" w597 {
                  tunnel: [w643 w644] -> w599
                  tunnel: w598 -> [w643 w645]
                  frame False {
                  }
                  frame True {
                    n316 = local read "Backlight"() -> (w646:i32[][])
                    n317 = Subtract(x=w645, y=w646) -> (x-y=w644:i32[][])
                  }
                }
                n318 = local read "滤波阈值"() -> (w592:dbl)
                n319 = local write "Data"(w598) -> ()
                n320 = local read "波长范围"() -> (w581:dbl[])
                n321 = Index Array(array=w599, index (row)=0 ("禁用的索引 (列)")) -> (element=w600:i32[])  [unwired: 1 in]
                n322 = Reverse 1D Array(array=w600) -> (reversed array=w582:i32[])
                n323 = call "转换至动态数据2"("Array"=w581) -> ("Dynamic Data Type"=w602:dynamicdata)  [unwired: 3 in]
                n324 = call "转换至动态数据"("Array"=w582) -> ("Dynamic Data Type"=w603:dynamicdata)  [unwired: 3 in]
                n325 = call "Build XY Graph2"("Y Input"=w603, "X Input"=w602) -> ("XY Graph"=w601:cluster{"Y":dbl[], "Y":dbl[]}[])  [unwired: 8 in, 1 out]
                n326 = local write "Spectrum"(w601) -> ()
                n327 = local read "X Pixels:"() -> (w588:i32)
                n328 = local read "滤波阈值"() -> (w586:dbl)
                n329 = call <vilib>:"Median Filter.vi"("left rank"=6, "X"=w582) -> ("Filtered X"=w587:dbl[])  [unwired: 8 in, 1 out]
                n330 = In Range and Coerce(upper limit=w592, x=w587, lower limit=-100.0) -> (In Range?=w591:bool[])  [unwired: 1 out]
                n331 = local write "范围内？"(w591) -> ()
                n332 = Not(x=w591) -> (.not. x?=w584:bool[])
                n333 = Or Array Elements(Boolean array=w584) -> (logical OR=w589:bool)
                n334 = case shown="真" w589 {
                  tunnel: w588 -> [_ w630]
                  tunnel: w587 -> [w626 w629]
                  tunnel: [w626 w628] -> w590
                  tunnel: w586 -> [_ w627]
                  frame False {
                  }
                  frame True {
                    n335 = for {
                      N: w630 -> [_]
                      tunnel: w629 -> [w634] mode=indexing
                      tunnel: [w633] -> w628 mode=indexing
                      shift-right: [w633] -> _
                      shift-left: _ -> [w632]
                      tunnel: w627 -> [w631]
                      n336 = Greater?(x=w634, y=w631) -> (0:w636:bool)
                      n337 = Less?(x=w634, y=-100.0) -> (x < y?=w637:bool)
                      n338 = Or(x=w636, y=w637) -> (x .or. y?=w635:bool)
                      n339 = case shown="真" w635 {
                        tunnel: w634 -> [w639 _]
                        tunnel: [w639 w641] -> w633
                        tunnel: w632 -> [_ w642]
                        frame False {
                        }
                        frame True {
                          n340 = call <vilib>:"Median Filter PtByPt.vi"("rank"=5, "x"=w642) -> ("Filtered x"=w641:dbl)  [unwired: 2 in, 1 out]
                        }
                      }
                    }
                  }
                }
                n341 = case shown="真" "是否拟合" {
                  tunnel: w590 -> [w612 w615]
                  tunnel: w581 -> [_ w614]
                  tunnel: [w612 w613] -> w594
                  frame False {
                  }
                  frame True {
                    n342 = call "转换至动态数据7"("Array"=w615) -> ("Dynamic Data Type"=w620:dynamicdata)  [unwired: 3 in]
                    n343 = call "转换至动态数据8"("Array"=w614) -> ("Dynamic Data Type"=w621:dynamicdata)  [unwired: 3 in]
                    n344 = call "曲线拟合2"("Locations"=w621, "Signals"=w620) -> ("best fit"=w618:dynamicdata, "non-linear coefficients"=w619:dynamicdata)  [unwired: 5 in, 3 out]
                    n345 = call "从动态数据转换3"("Dynamic Data Type"=w619) -> ("Array"=w622:dbl[])  [unwired: 3 in]
                    n346 = call "从动态数据转换4"("Dynamic Data Type"=w618) -> ("Array"=w613:dbl[])  [unwired: 3 in]
                    n347 = Index Array(array=w622, index #1=0 ("索引"), index #2=1 ("索引")) -> (element #1=w624:dbl, element #2=w623:dbl)
                    n348 = local write "拟合参数"(w622) -> ()
                    n349 = Build Array(w615, w613) -> (w625:dbl[][])
                    n350 = local write "xc"(w624) -> ()
                    n351 = local write "best fit"(w625) -> ()
                    n352 = local write "w"(w623) -> ()
                  }
                }
                n353 = Build Array(w581, w582, w594) -> (w580:dbl[][])
              }
              frame #4 {
                n354 = case shown="真" "是否保存" {
                  tunnel: w647 -> [_ w651]
                  frame False {
                  }
                  frame True {
                    n355 = Get Date/Time In Seconds() -> (seconds since 1Jan1904=w665:timestamp)
                    n356 = Get Date/Time String(date format (0)=enum16{"short", "long", "abbreviated"}."abbreviated" ("日期格式(0)"), seconds (now)=w665, want seconds? (F)=TRUE ("需要秒？(F)")) -> (date string=w663:string, time string=w664:string)
                    n357 = Search and Replace String(replace all?=TRUE ("替换全部？(F)"), input string=w664, search string=":" ("搜索字符串"), replace string="-" ("替换字符串(\"\")")) -> (result string=w662:string)  [unwired: 4 in, 3 out]
                    n358 = local read "最终存储路径 2"() -> (w666:path)
                    n359 = Path To String(path=w666) -> (string=w669:string)
                    n360 = Concatenate Strings(w669, w663, w662, "光谱" ("字符串"), ".xls" ("字符串")) -> (w668:string)
                    n361 = String To Path(string=w668) -> (path=w667:path)
                    n362 = call-poly <vilib>:"Write Delimited Spreadsheet.vi"("file path (dialog if empty)"=w667, "format (%.3f)"="%.16f", "2D data"=w651, "append to file? (new file:F)"=TRUE ("append to file? (F)"), "transpose? (no:F)"=TRUE ("transpose? (F)")) -> ()  [unwired: 9 in, 2 out]
                  }
                }
                n363 = case shown="真" "Save Backlight" {
                  frame False {
                  }
                  frame True {
                    w670 = TRUE ("删除背景光")
                    n364 = local read "Data"() -> (w672:i32[][])
                    n365 = local write "Backlight"(w672) -> ()
                    n366 = local write "cut backlight"(w670) -> ()
                    n367 = local write "backlight"(w670) -> ()
                    n368 = local write "Save Backlight"(FALSE ("Save Backlight")) -> ()
                  }
                }
                n369 = local write "CCD Busy"(FALSE ("CCD Busy")) -> ()
              }
            }
          }
        }
        n370 = case shown="真" "Setup" {
          tunnel: w516 -> [_ w686]
          tunnel: w517 -> [_ w685]
          frame False {
          }
          frame True {
            n371 = stacked-sequence {
              tunnel: w686 -> [_ w700 _]
              tunnel: w685 -> [_ w688 _]
              frame #0 {
                n372 = local write "indicator"("Setting up the detector" ("indicator")) -> ()
              }
              frame #1 {
                w698 = 1 items=["JYMCD_ACQ_FORMAT_IMAGE", "JYMCD_ACQ_FORMAT_SCAN"] ("Acquisition type")
                n373 = local read "Gain Number"() -> (w693:i32[])
                n374 = local read "GAIN"() -> (w689:u16)
                n375 = local read "ADC Number"() -> (w694:i32[])
                n376 = local read "ADC"() -> (w690:u16)
                n377 = Index Array(array=w693, index=w689) -> (element=w691:i32)
                n378 = Index Array(array=w694, index=w690) -> (element=w692:i32)
                n379 = local read "Number of Areas :"() -> (w696:u16)
                n380 = local read "areas :"() -> (w697:i32[][])
                n381 = call "Setup CCD.vi"("numAreas"=w696, "areas :"=w697, "JYCCDLib.IJYCCDReqd"=w688, "entrée d'erreur (pas d'erreur)"=w700, "Acquisition type"=w698, "Gain"=w691, "Select ADC"=w692, "Integration time(ms)"="Integration time (ms) :") -> ("DataSize"=→"DataSize":i32)  [unwired: 1 out]
                "JYCCDLib.IJYCCDReqd" <- w688
              }
              frame #2 {
                w701 = TRUE ("Visible")
                n382 = property on="Continuous" class="Bool (严格)"("Visible"=w701) -> ()  [unwired: 2 in, 2 out]
                n383 = property on="Acquire" class="Bool"("Visible"=w701) -> ()  [unwired: 2 in, 2 out]
                n384 = local write "indicator"("Ready !" ("indicator")) -> ()
              }
            }
          }
        }
        n385 = case shown="真" "Temperature" {
          tunnel: w517 -> [_ w675]
          tunnel: w516 -> [_ w674]
          frame False {
            n386 = property on="temp graph" class="WFChart (严格)"("Visible"=FALSE) -> ()  [unwired: 2 in, 2 out]
          }
          frame True {
            n387 = stacked-sequence {
              tunnel: w675 -> [_ w680]
              tunnel: w674 -> [_ w679]
              frame #0 {
                n388 = property on="temp graph" class="WFChart (严格)"("Visible"=TRUE) -> ()  [unwired: 2 in, 2 out]
              }
              frame #1 {
                w678 = u16 0 items=["° Celsius", "Kelvin", "° Farenheit"] ("units")
                n389 = call "read temperature.vi"("entrée d'erreur (pas d'erreur)"=w679, "units"=w678, "JYCCDLib.IJYCCDReqd"=w680) -> ("Current Temperature"=w677:dbl)
                n390 = local write "temp graph"(w677) -> ()
              }
            }
          }
        }
        n391 = Wait Until Next ms Multiple(millisecond multiple=u32 50 ("n millisecondes")) -> ()  [unwired: 1 out]
      }
    }
    frame #7 {
      n392 = Close Reference(reference=w704, error in (no error)=w703) -> ()  [unwired: 1 out]
    }
  }
  n393 = stacked-sequence {
    seq-local: [_ _ w714 _ _] -> [_ _ _ w724 w729]
    seq-local: [_ _ w713 _ _] -> [_ _ _ w723 _]
    seq-local: [_ _ _ w722 _] -> [_ _ _ _ _]
    frame #0 {
      n394 = call "Get Monos From Config Browser.vi"() -> ("UniqueIDs"=w709:string[], "Mono ID"=w710:string[])  [unwired: 3 in, 1 out]
      n395 = Build Cluster Array(w710, w709) -> (w707:cluster{"String":string, "String":string}[])
      n396 = property on="Mono ID" class="CmbBox"("Strings And Values []"=w707) -> ()  [unwired: 2 in, 2 out]
      n397 = Index Array(array=w707, index=0) -> (element=w708:cluster{"String":string, "String":string})
      n398 = Unbundle(w708) -> ("String"=w705:string)  [unwired: 1 out]
      "Current UniqueID" <- w705
      n399 = local write "Mono ID"(w705) -> ()
    }
    frame #1 {
      n400 = while {
        stop <- "Connect" stop-if-true
        n401 = local read "Mono ID"() -> (w711:string)
        n402 = local write "Current UniqueID"(w711) -> ()
      }
    }
    frame #2 {
      n403 = local read "Mono ID"() -> (w716:string)
      n404 = call "JYInitMono.vi"("Unique ID"=w716, "Force Init"="Force\nInitialization") -> ("Refnum out"=w714:refnum<k7>, "Initialized"=→"Initialized JY":bool, "error out"=w713:errorcluster)  [unwired: 9 in, 2 out]
    }
    frame #3 {
      n405 = call "Show Current Grating.vi"("Refnum in"=w724, "error in (no error)"=w723) -> ("Gratings"=w725:dbl[], "Grating Index"=w719:i32, "Current Grating"=w721:dbl, "Current Description"=w718:string, "error out"=w722:errorcluster)  [unwired: 5 in, 4 out]
      "Gratings" <- w725
      n406 = local write "Current Grating"(w721) -> ()
      n407 = local write "Current Description"(w718) -> ()
      n408 = Number To Decimal String(number=w725) -> (decimal integer string=w727:string[])  [unwired: 1 in]
      n409 = Number To Decimal String(number=w719) -> (decimal integer string=w720:string)  [unwired: 1 in]
      n410 = property on="Target Grating" class="CmbBox"("Value"=w720) -> ()  [unwired: 2 in, 2 out]
      n411 = Build Cluster Array(w727, string[] ["1", "2", "3"]) -> (w728:cluster{"Numeric":string, string}[])
      n412 = property on="Target Grating" class="CmbBox"("Strings And Values []"=w728) -> ()  [unwired: 2 in, 2 out]
    }
    frame #4 {
      n413 = while {
        tunnel: w729 -> [w731]
        stop <- w730 stop-if-true
        n414 = stacked-sequence {
          seq-local: [w735 _ _ _ _] -> [_ w742 w753 _ w761]
          seq-local: [w734 _ _ _ _] -> [_ w741 w752 _ _]
          seq-local: [_ w740 _ _ _] -> [_ _ _ _ _]
          seq-local: [_ w739 _ _ _] -> [_ _ _ _ _]
          seq-local: [_ _ w745 _ _] -> [_ _ _ _ _]
          seq-local: [_ _ w744 _ _] -> [_ _ _ w755 _]
          tunnel: w731 -> [w733 _ _ w756 _]
          frame #0 {
            n415 = call "Show Current Grating.vi"("Refnum in"=w733) -> ("Grating Index"=→"Grating Index":i32, "Current Grating"=→"Current Grating":dbl, "Current Description"=→"Current Description":string, "error out"=w734:errorcluster, "JYMONOLib.IJYMonoReqd"=w735:refnum<k7>)  [unwired: 6 in, 4 out]
          }
          frame #1 {
            n416 = call "JYGetCurrentWL.vi"("error in (no error)"=w741, "JYMONOLib.IJYMonoReqd"=w742) -> ("error out"=w739:errorcluster, "Units"=→"Units":string, "Current WL"=→"Current WL":dbl, "JYMONOLib.IJYMonoReqd 2"=w740:refnum<k7>)  [unwired: 6 in]
          }
          frame #2 {
            w750 = u16 1 items=["Entrance", "Exit"] ("Mirror Number")
            w751 = u16 0 items=["Entrance", "Exit"] ("Mirror Number")
            n417 = call "JYGetMirrorPos.vi"("error in (no error)"=w752, "Mirror"=w751, "Refnum In"=w753) -> ("error out"=w748:errorcluster, "Current Mirror Position"=→"Entrance Mirror\nPosition":i32, "Refnum Out"=w749:refnum<k7>)  [unwired: 1 in]
            n418 = call "JYGetMirrorPos.vi"("error in (no error)"=w748, "Mirror"=w750, "Refnum In"=w749) -> ("error out"=w744:errorcluster, "Current Mirror Position"=→"Exit Mirror\nPosition":i32, "Refnum Out"=w745:refnum<k7>)  [unwired: 1 in]
          }
          frame #3 {
            w758 = u16 0 items=["Front Entrance", "Side Entrance", "Front Exit", "Side Exit", "First Intermediate", "Second Intermediate"] ("Slit")
            n419 = call "JYGetSlits.vi"("MonoRefNum IN"=w756, "Slit"=w758, "error in (no error)"=w755) -> ("Units"=→"Units 2":string, "Slit Width"=→"Front Entrance":dbl, "error out"=→"error out":errorcluster)  [unwired: 13 in, 1 out]
          }
          frame #4 {
            n420 = case shown="真" "Move To\nTarget Positions" {
              tunnel: w761 -> [_ w762]
              frame False {
              }
              frame True {
                n421 = stacked-sequence {
                  seq-local: [w764 _ _ _] -> [_ w770 _ _]
                  seq-local: [_ w768 _ _] -> [_ _ w785 _]
                  seq-local: [_ _ w772 _] -> [_ _ _ w791]
                  seq-local: [_ _ _ w788] -> [_ _ _ _]
                  tunnel: w762 -> [w766 w769 w783 w792]
                  frame #0 {
                    n422 = property on="Target Grating" class="CmbBox"() -> ("Value"=w763:string)  [unwired: 2 in, 2 out]
                    n423 = local read "error out"() -> (w765:errorcluster)
                    n424 = Decimal String To Number(string=w763) -> (number=w767:i32)  [unwired: 2 in, 1 out]
                    n425 = call "JYTurret.vi"("error in (no error)"=w765, "Grating Index"=w767, "JYMONOLib.IJYMonoReqd"=w766) -> ("error out"=w764:errorcluster)  [unwired: 2 out]
                  }
                  frame #1 {
                    # "Move Grating to Target Position"
                    n426 = call "JYMoveToWavelength.vi"("error in (no error)"=w770, "Target WL"="Target WL", "RefNum In"=w769) -> ("error out"=w768:errorcluster)  [unwired: 1 in, 2 out]
                  }
                  frame #2 {
                    w778 = u16 1 items=["Entrance", "Exit"] ("Mirror Number")
                    w777 = u16 0 items=["Entrance", "Exit"] ("Mirror Number")
                    w784 = u16 1 items=["Entrance", "Exit", "Front", "Side"] ("Mirror Number")
                    w787 = u16 0 items=["Entrance", "Exit", "Front", "Side"] ("Mirror Number")
                    # "Move Mirrors"
                    n427 = call "JYMirrorMove.vi"("error in (no error)"=w785, "Mirror Position"="Entrance Mirror", "Mirror Number"=w787, "RefNum In"=w783) -> ("error out"=w782:errorcluster)  [unwired: 6 in, 1 out]
                    n428 = call "JYMirrorMove.vi"("error in (no error)"=w782, "Mirror Position"="Exit Mirror", "Mirror Number"=w784, "RefNum In"=w783) -> ("error out"=w775:errorcluster, "MonoRefNum Out"=w776:refnum<k7>)  [unwired: 6 in]
                    n429 = call "JYGetMirrorPos.vi"("error in (no error)"=w775, "Mirror"=w777, "Refnum In"=w776) -> ("error out"=w780:errorcluster, "Current Mirror Position"=w774:i32, "Refnum Out"=w779:refnum<k7>)  [unwired: 1 in]
                    n430 = local write "Entrance Mirror\nPosition"(w774) -> ()
                    n431 = call "JYGetMirrorPos.vi"("error in (no error)"=w780, "Mirror"=w778, "Refnum In"=w779) -> ("error out"=w772:errorcluster, "Current Mirror Position"=w773:i32)  [unwired: 1 in, 1 out]
                    n432 = local write "Exit Mirror\nPosition"(w773) -> ()
                  }
                  frame #3 {
                    w790 = u16 0 items=["Front Entrance", "Side Entrance", "Front Exit", "Side Exit", "First Intermediate", "Second Intermediate"] ("Slit")
                    # "Set New Slit Positions"
                    n433 = call "JYSlits.vi"("JYMONOLib.IJYMonoReqd"=w792, "Slit"=w790, "error in (no error)"=w791, "Slit Width"="Target\nFront Entrance") -> ("error out"=w788:errorcluster)  [unwired: 1 in, 1 out]
                  }
                }
              }
            }
          }
        }
        n434 = local read "Close"() -> (w730:bool)
      }
    }
  }
  n435 = flat-sequence {
    frame #0 {
      n436 = call <vilib>:"Create Report.vi"("window state (normal)"=T3."no change", "report type"=Report_Type."Excel", "template (empty)"=path "D:/desktop/train/TEST1/Save/2670中心波长.xlsx") -> ("report out"=w799:refnum<class "NI_report.lvclass">, "error out"=w798:errorcluster)  [unwired: 11 in]
      n437 = call-poly <vilib>:"Excel Get Data.vi"("report in"=w799, "data type"=string[][] [], "error in (no error)"=w798) -> ("report out"=w794:refnum<class "NI_report.lvclass">, "data"=w802:string[][], "error out"=w793:errorcluster)  [unwired: 10 in]
      n438 = call-dynamic "Dispose Report.vi"("report in"=w794, "error in (no error)"=w793) -> ()  [unwired: 13 in, 1 out]
      n439 = Index Array(array=w802, index (col)=0 ("禁用的索引 (列)")) -> (element=w804:string[])  [unwired: 1 in]
      n440 = Fract/Exp String To Number(string=w804) -> (number=→"波长范围":dbl[])  [unwired: 3 in, 1 out]
    }
  }
